vi "Autonomous Independent.vi"() -> ()   [LabVIEW 2020]
doc: "This VI is called when autonomous begins, and will automatically be terminated when autonomous ends. You can carry out timed or sensor driven robot movement independently without needing to return to the caller."
uses:
  <vilib>/Rock Robotics/WPI/ThirdParty/Phoenix-LabVIEW/Motor Controller/Controls/CTRE_Phoenix_MotorControl_ControlMode.ctl
  <vilib>/Rock Robotics/WPI/Solenoid/WPI_SolenoidValue.ctl
  <vilib>/Rock Robotics/WPI/Utilities/WPI_GetSetVariantRefNum.vi
  <vilib>/Rock Robotics/Network Tables/NT Read String.vi
  <vilib>/Rock Robotics/Network Tables/NT Write Numeric Array.vi
  <vilib>/Rock Robotics/WPI/Solenoid/WPI_SolenoidSetEnum.vi
  <vilib>/Rock Robotics/Network Tables/NT Read Number.vi
  AutonBoolean.vi
panel:
  out "Ty 24":dbl
  out "Ty 23":dbl
  out "Ty 22":dbl
  out "Ty 21":dbl
  out "Ty 20":dbl
  out "Ty 19":dbl
  out "Ty 18":dbl
  out "Ty 17":dbl
  out "Orange Limit Pressed 10":bool
  out "Blue Limit Pressed 10":bool
  out "Ty 16":dbl
  out "Orange Limit Pressed 9":bool
  out "Blue Limit Pressed 9":bool
  out "Ty 15":dbl
  out "Intake 5":bool
  out "Elevate 5":bool
  out "Ty 14":dbl
  out "Ty 13":dbl
  out "Ty 12":dbl
  out "Ty 11":dbl
  out "Ty 10":dbl
  out "Ty 9":dbl
  out "Orange Limit Pressed 4":bool
  out "Blue Limit Pressed 4":bool
  out "Ty 4":dbl
  out "Orange Limit Pressed 3":bool
  out "Blue Limit Pressed 3":bool
  out "Ty 3":dbl
  out "Intake 2":bool
  out "Elevate 2":bool
  out "Intake":bool
  out "Elevate":bool
  out "Orange Limit Pressed":bool
  out "Blue Limit Pressed":bool
  out "Ty":dbl
  out "Orange Limit Pressed 2":bool
  out "Blue Limit Pressed 2":bool
  out "Ty 2":dbl
  out "Intake 3":bool
  out "Elevate 3":bool
  out "Orange Limit Pressed 5":bool
  out "Blue Limit Pressed 5":bool
  out "Ty 5":dbl
  out "Orange Limit Pressed 6":bool
  out "Blue Limit Pressed 6":bool
  out "Ty 6":dbl
  out "Intake 4":bool
  out "Elevate 4":bool
  out "Orange Limit Pressed 7":bool
  out "Blue Limit Pressed 7":bool
  out "Ty 7":dbl
  out "Orange Limit Pressed 8":bool
  out "Blue Limit Pressed 8":bool
  out "Ty 8":dbl
  # "Be sure to right-click and choose Data Operations>>Make Current Value default if you want to save the array values with the VI"
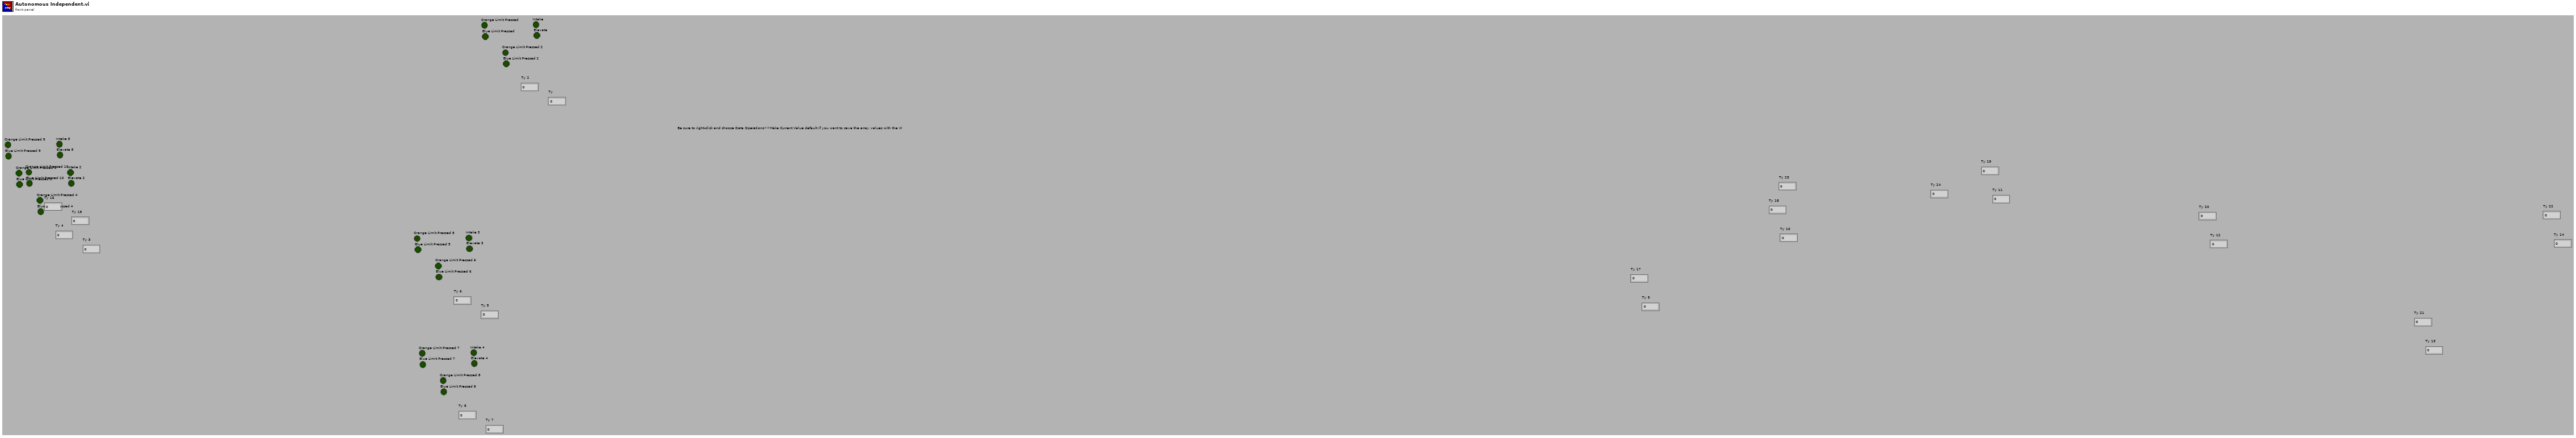
[diagram p1: front panel]
types:
  T1 = typedef "WPI_JoystickDevRef.ctl" = cluster{"Device":T2}
  T2 = typedef "WPI_JoystickDeviceEnum.ctl" = enum16{"USB 0", "USB 1", "USB 2", "USB 3", "USB 4", "USB 5"}
  T3 = typedef "WPI_SolenoidValue.ctl" = enum16{"Off", "On", "Forward", "Reverse"}
  T4 = typedef "WPI_SwitchDevRef.ctl" = cluster{"DevStatus":errorcluster, "DIO Channel":T5, "CntIndex":T6, "Normally Closed":bool}
  T5 = typedef "FPGA_DIOChannel.ctl" = enum8{"DIO 0", "DIO 1", "DIO 2", "DIO 3", "DIO 4", "DIO 5", "DIO 6", "DIO 7", "DIO 8", "DIO 9", "DIO MXP 0", "DIO MXP 1", "DIO MXP 2", "DIO MXP 3", "DIO MXP 4", "DIO MXP 5", "DIO MXP 6", "DIO MXP 7", "DIO MXP 8", "DIO MXP 9", "DIO MXP 10", "DIO MXP 11", "DIO MXP 12", "DIO MXP 13", "DIO MXP 14", "DIO MXP 15", "SPI Port CS1", "SPI Port CS2", "SPI Port CS3", "SPI Port MISO", "SPI Port MOSI", "Invalid"}
  T6 = typedef "FPGA_CounterCtrSystemIndex.ctl" = enum8{"Ctr 0", "Ctr 1", "Ctr 2", "Ctr 3", "Ctr 4", "Ctr 5", "Ctr 6", "Ctr 7", "Invalid"}
  T7 = typedef "WPI_SolenoidDevRef.ctl" = cluster{"DevStatus":errorcluster, "Pneumatics Control Module":u8, "Forward Solenoid Channel":T8, "Reverse Solenoid Channel":T8}
  T8 = typedef "WPI_SolenoidChannel.ctl" = enum8{"Solenoid 0", "Solenoid 1", "Solenoid 2", "Solenoid 3", "Solenoid 4", "Solenoid 5", "Solenoid 6", "Solenoid 7", "Solenoid 8", "Solenoid 9", "Solenoid 10", "Solenoid 11", "Solenoid 12", "Solenoid 13", "Solenoid 14", "Solenoid 15", "Invalid"}
  T9 = typedef "WPI_MotorControlDeviceRef.ctl" = cluster{"DeviceStatus":errorcluster, "Type":T10, "PWM":cluster{"PWM Channel":T11, "DeadBand":T12}, "CAN":cluster{"Device Number":u8, "SetOutput VI Ref":variant, "GetOutput VI Ref":variant, "Enable VI Ref":variant, "Disable VI Ref":variant, "Data":variant}, "Invert":bool, "DIO PWM":cluster{"PWM \"Enable\" Channel":T11, "DIOChannel":T5, "PWM Rate":dbl}}
  T10 = typedef "WPI_MotorControlType.ctl" = enum16{"PWM", "CAN", "DIO PWM"}
  T11 = typedef "FPGA_DIOPWMChannel.ctl" = enum8{"PWM 0", "PWM 1", "PWM 2", "PWM 3", "PWM 4", "PWM 5", "PWM 6", "PWM 7", "PWM 8", "PWM 9", "PWM MXP 0", "PWM MXP 1", "PWM MXP 2", "PWM MXP 3", "PWM MXP 4", "PWM MXP 5", "PWM MXP 6", "PWM MXP 7", "PWM MXP 8", "PWM MXP 9", "Invalid"}
  T12 = typedef "WPI_PWMDeadband.ctl" = cluster{"Name":string, "maxPositivePwm":i32, "minPositivePwm":i32, "centerPwm":i32, "maxNegativePwm":i32, "minNegativePwm":i32, "angularRange":u16}
  T13 = typedef "CTRE_Phoenix_MotorControl_ControlMode.ctl" = u16
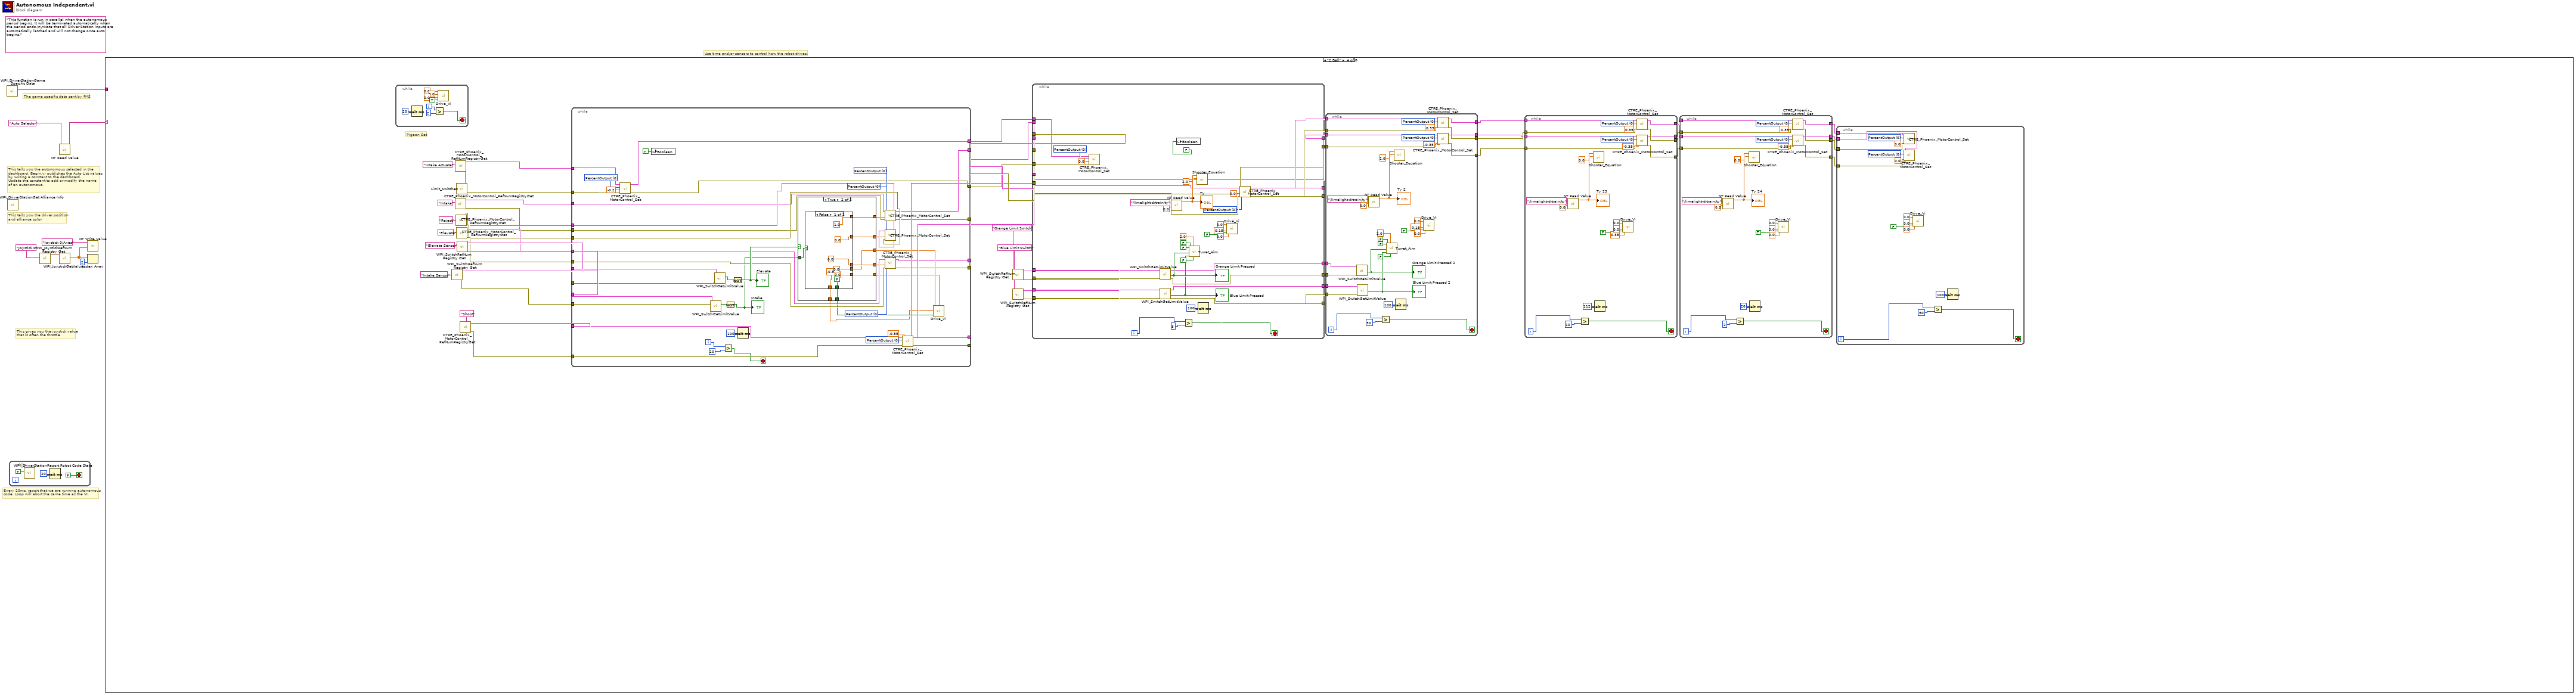
[diagram p0: block diagram]
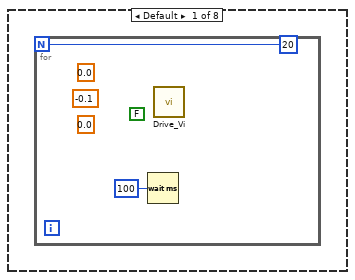
[diagram p2: hidden frame]
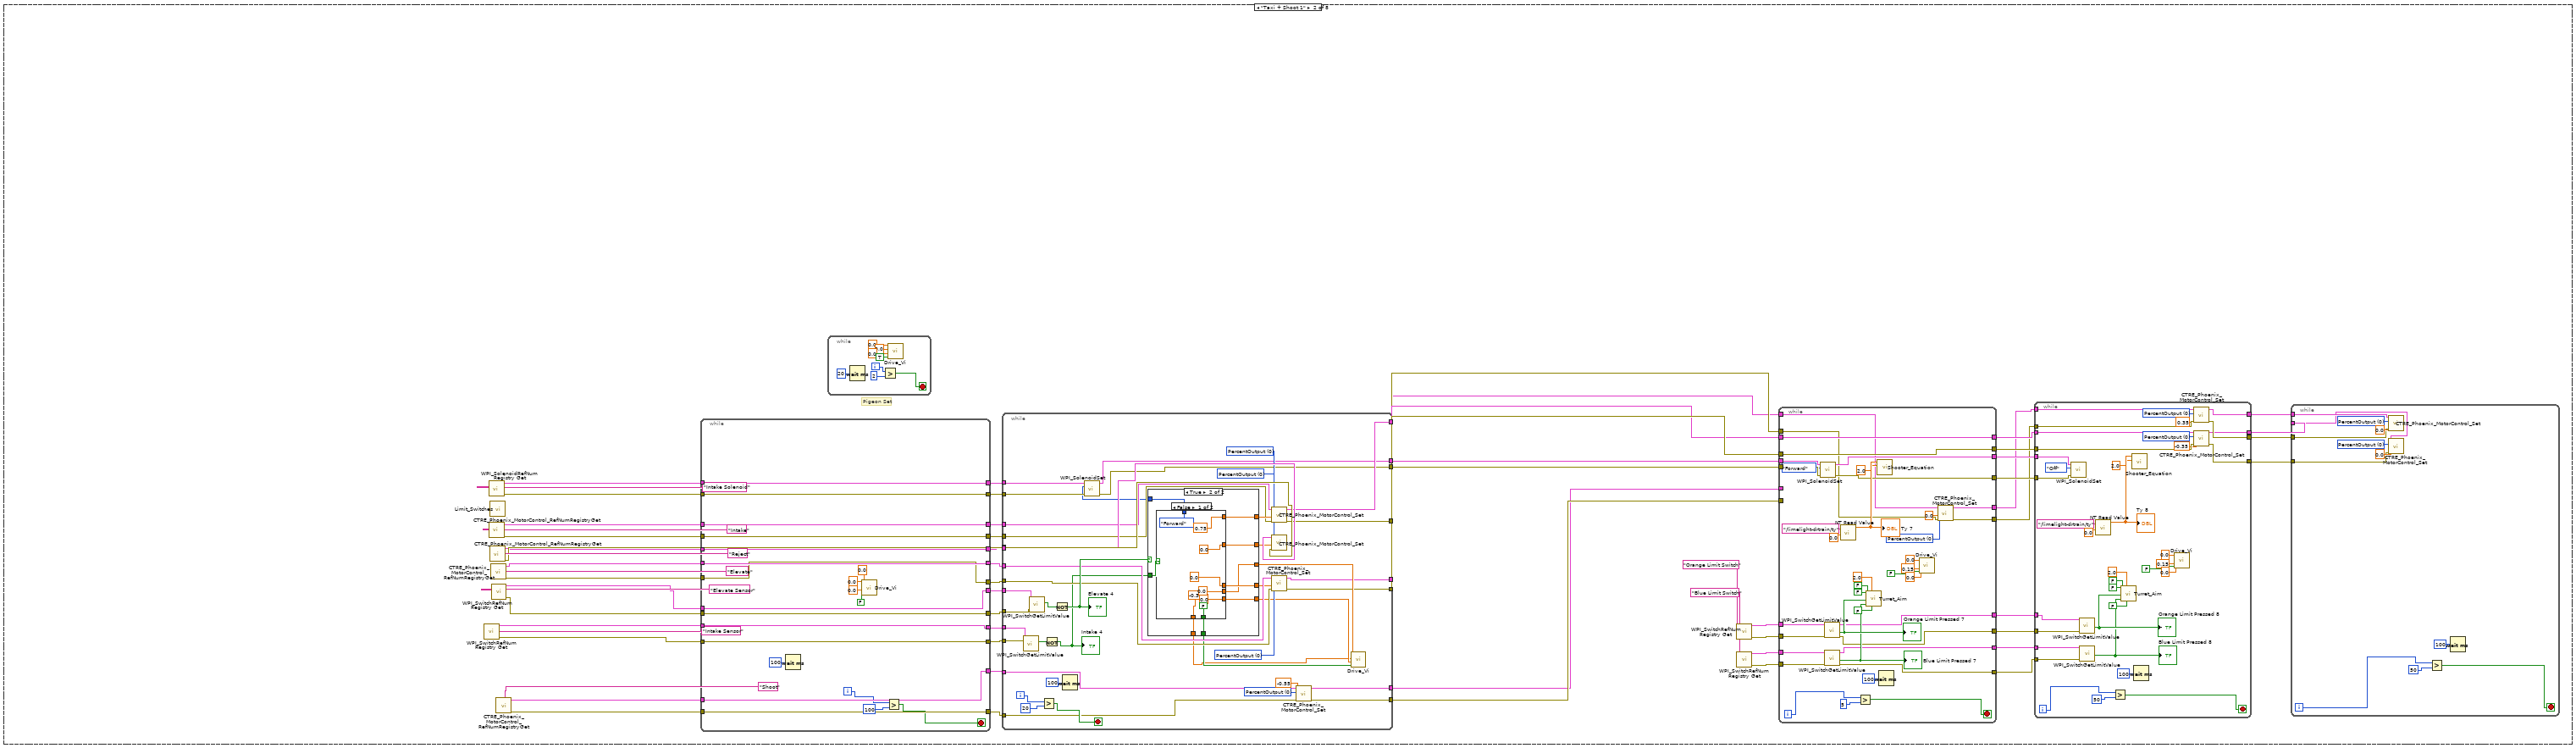
[diagram p3: hidden frame]
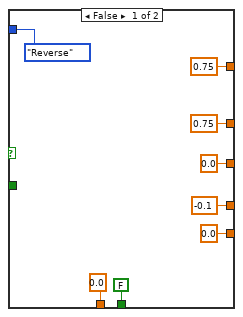
[diagram p4: hidden frame]
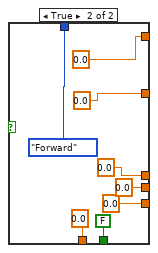
[diagram p5: hidden frame]
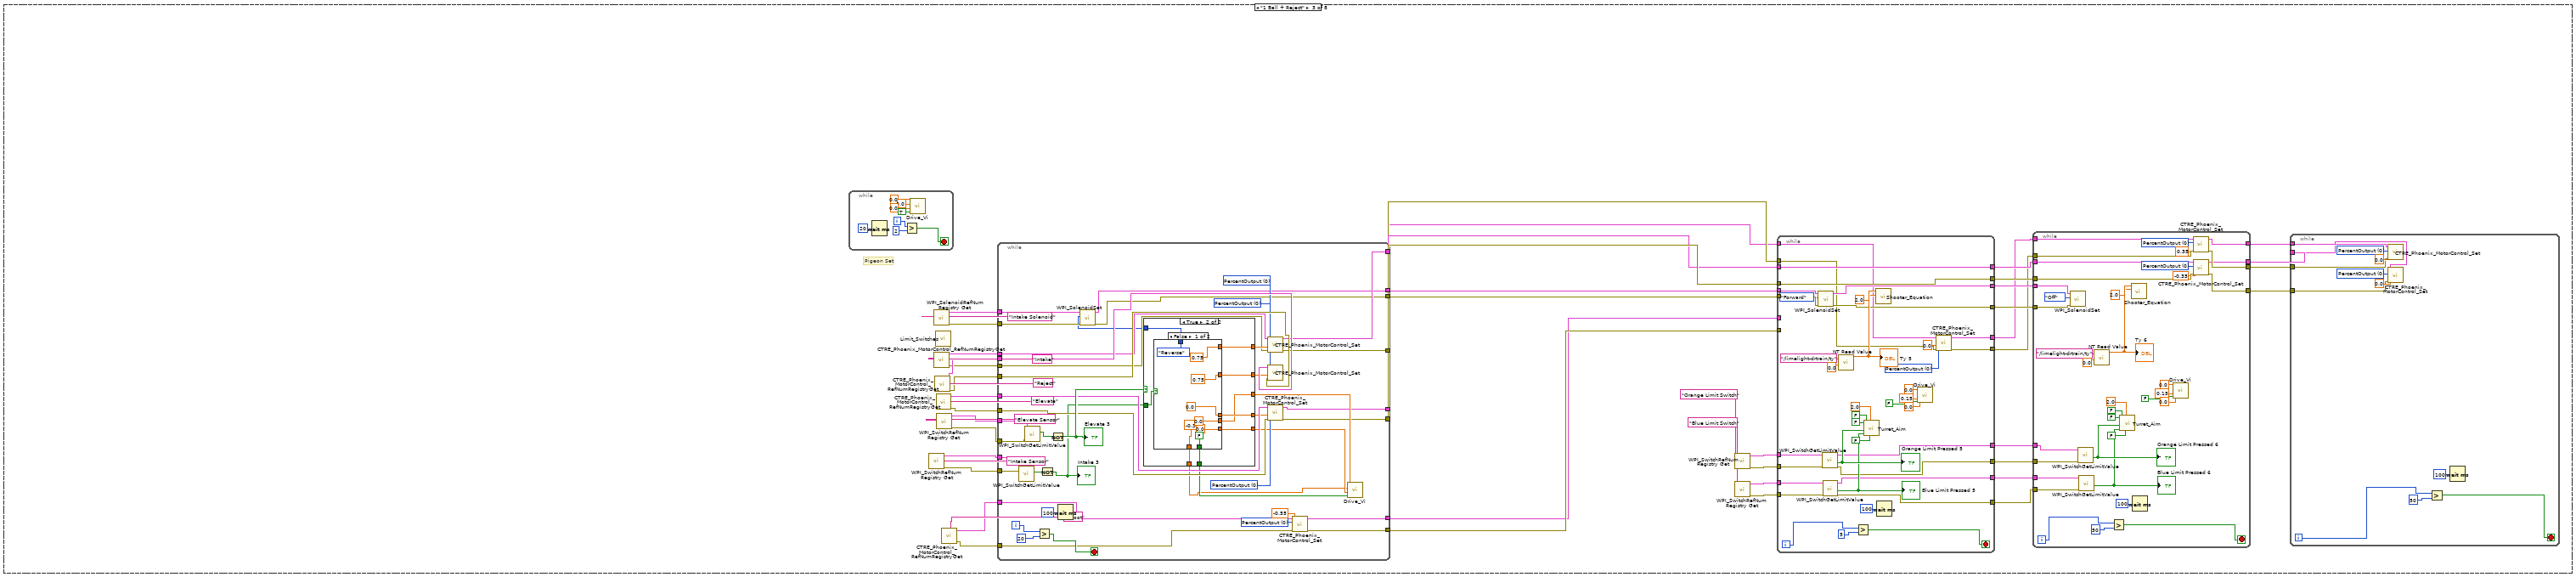
[diagram p6: hidden frame]
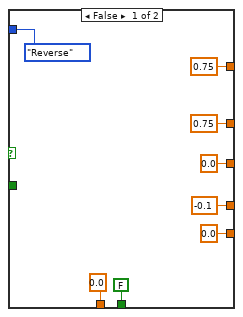
[diagram p7: hidden frame]
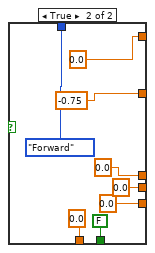
[diagram p8: hidden frame]
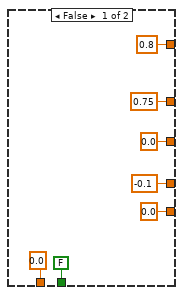
[diagram p9: hidden frame]
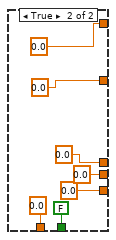
[diagram p10: hidden frame]
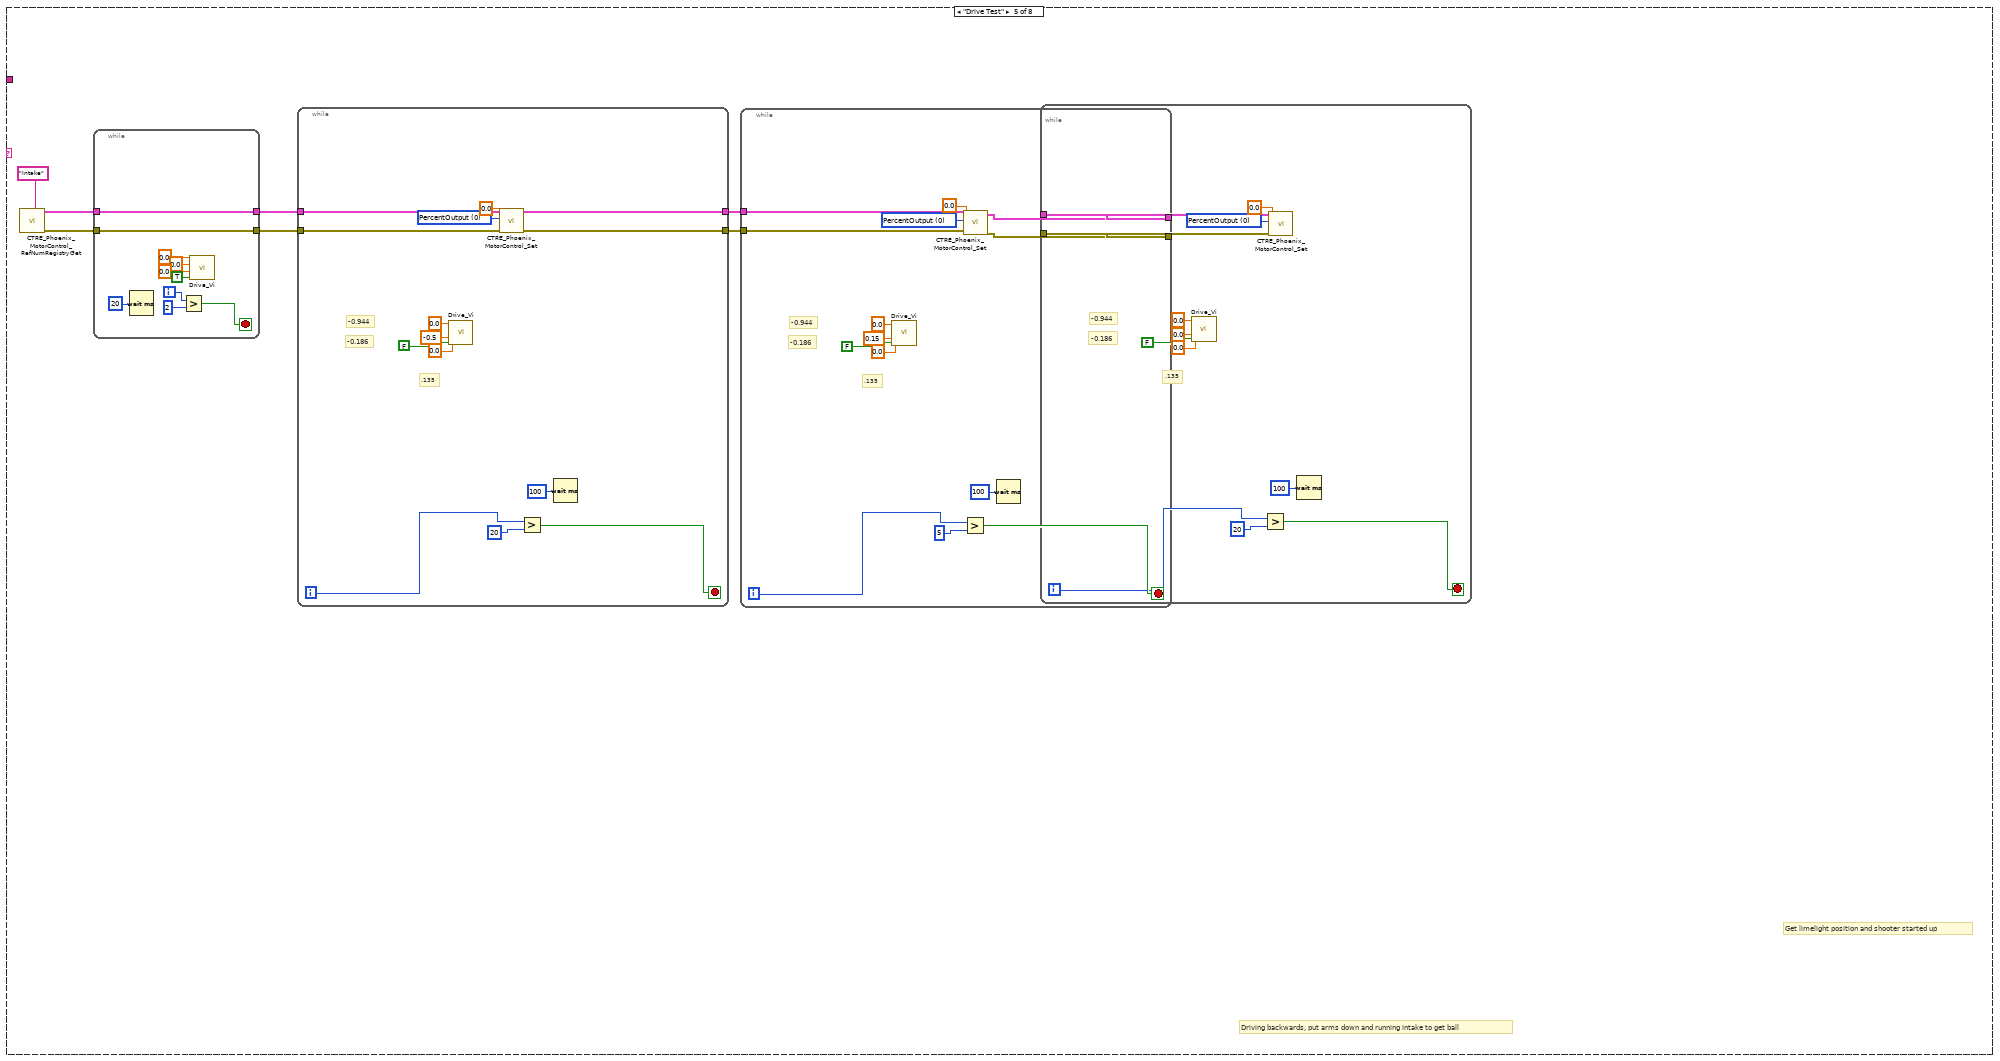
[diagram p11: hidden frame]
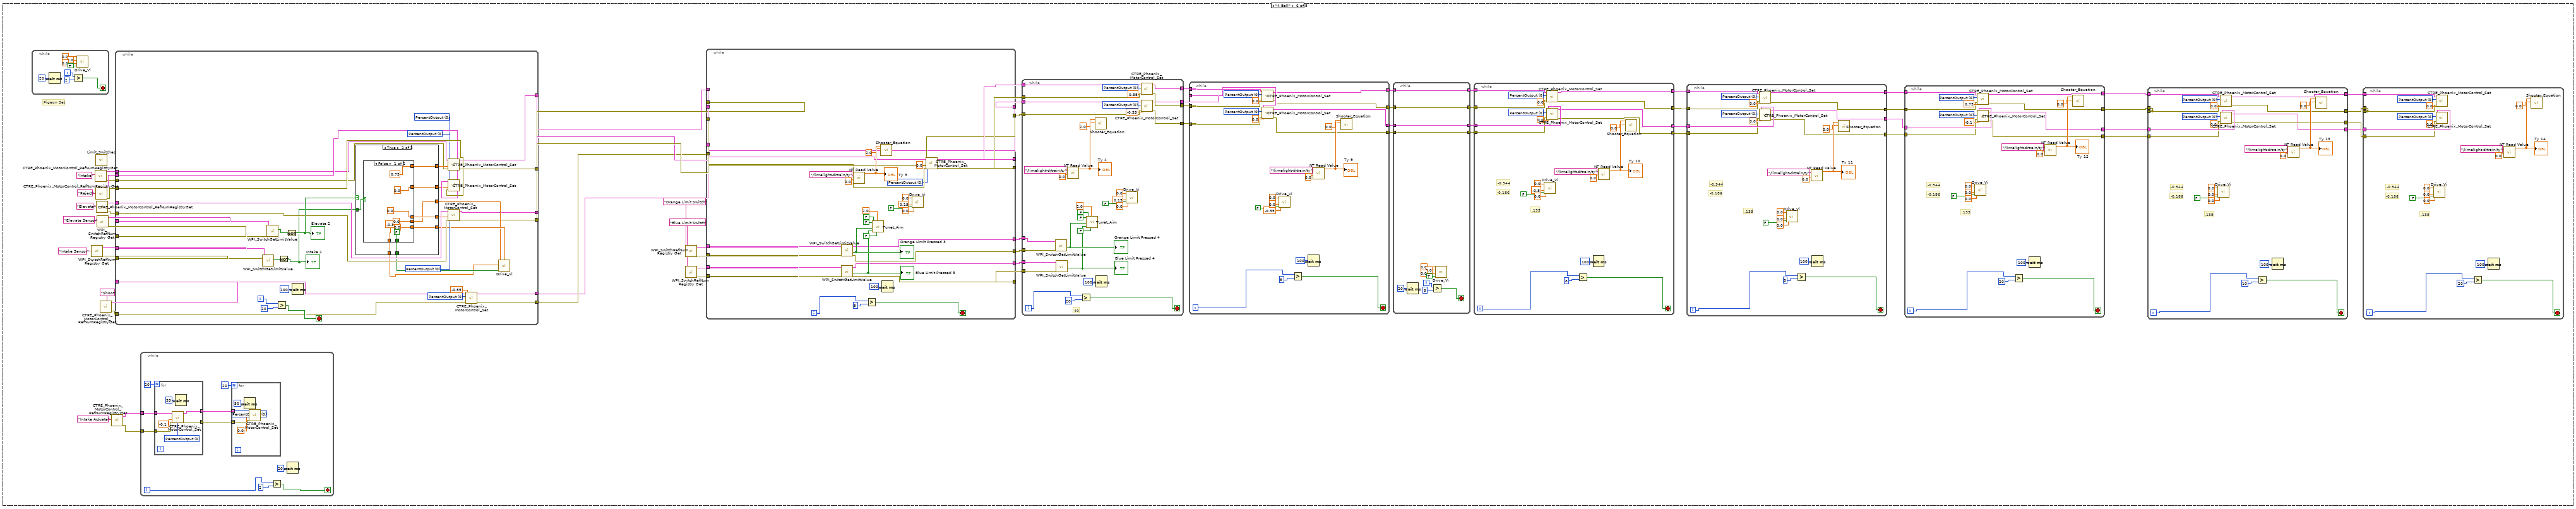
[diagram p12: hidden frame]
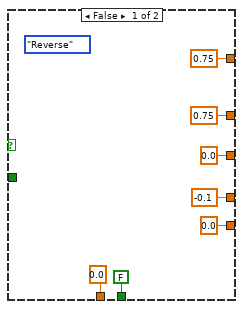
[diagram p13: hidden frame]
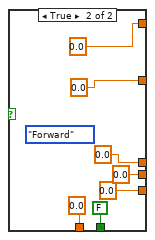
[diagram p14: hidden frame]
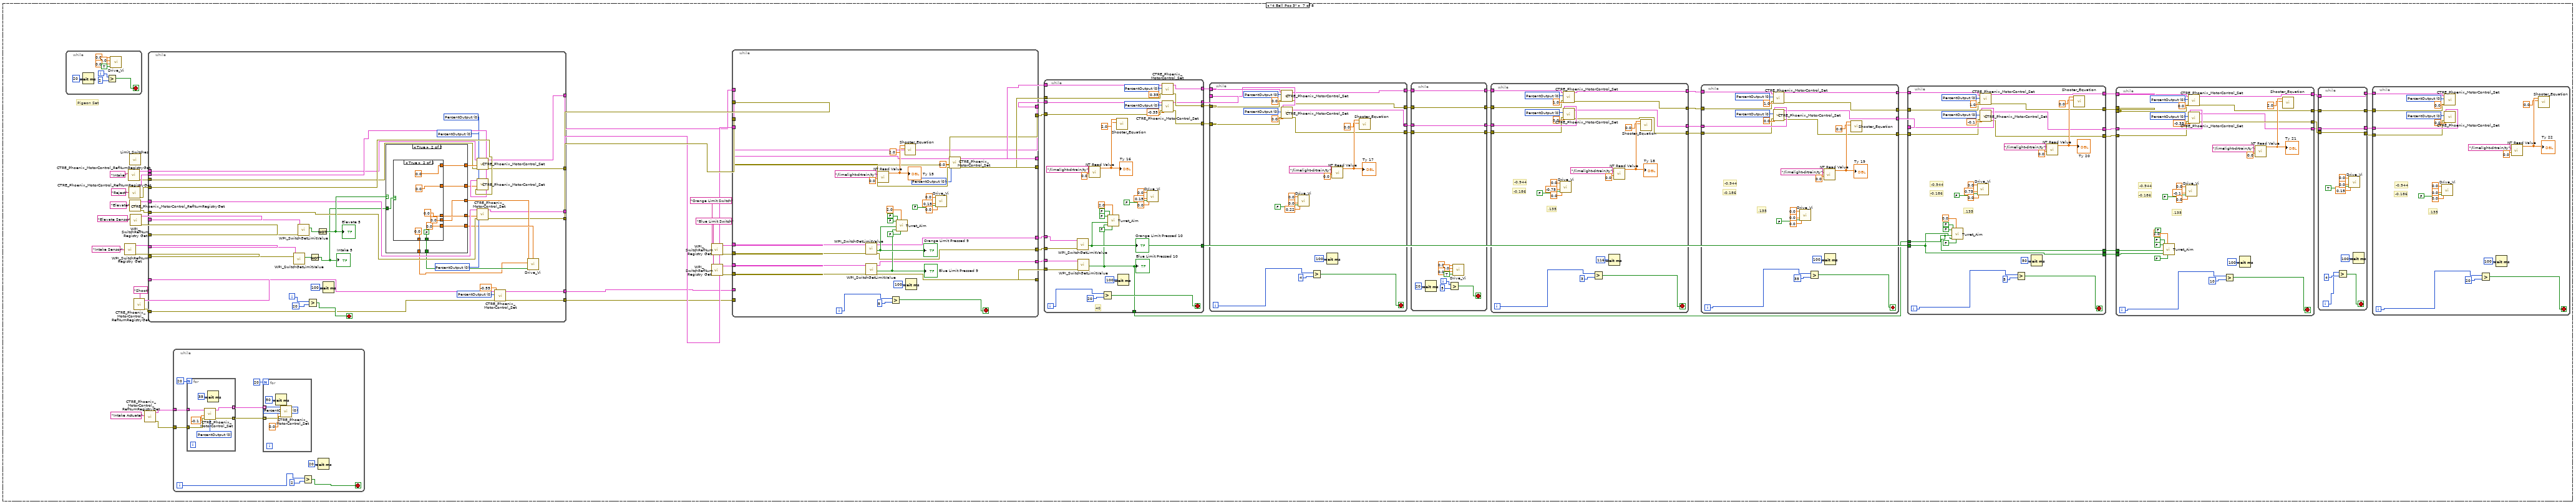
[diagram p15: hidden frame]
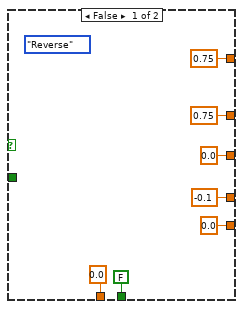
[diagram p16: hidden frame]
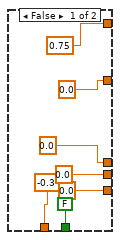
[diagram p17: hidden frame]
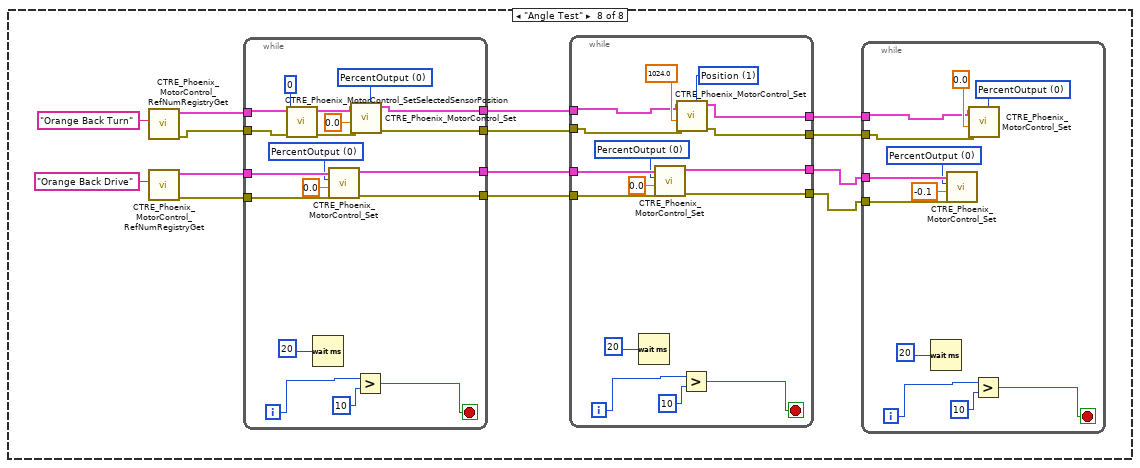
[diagram p18: hidden frame]
diagram:
  (unwired) "This function is run in parallel when the autonomous period begins. It will be terminated automatically when the period ends.\n\nNote that all Driver Station inputs are automatically latched and will not change once auto begins."
  # "The game specific data sent by FMS"
  # "This tells you the autonomous selected in the \ndashboard. Begin.vi publishes the Auto List values\nby writing a constant to the dashboard.\nUpdate the constant to add or modify the name\nof an autonomous."
  # "Every 20ms, report that we are running autonomous\ncode. Loop will abort the same time as the VI."
  # "This gives you the joystick value\nthat is often the throttle"
  # "Use time and/or sensors to control how the robot drives."
  # "This tells you the driver position\nand alliance color"
  n1 = call <vilib>:"WPI_DriverStationGame Specific Data.vi"() -> ("Game Specific Data"=w1:string)  [unwired: 11 in]
  n2 = call <vilib>:"WPI_DriverStationGet Alliance Info.vi"() -> ()  [unwired: 12 out]
  n3 = while {
    stop <- FALSE stop-if-true
    n4 = call <vilib>:"WPI_DriverStationReport Robot Code State.vi"("Autonomous"=TRUE) -> ()  [unwired: 10 in, 1 out]
    n5 = Wait (ms)(milliseconds to wait=u32 20) -> ()  [unwired: 1 out]
  }
  n6 = call <vilib>:"WPI_JoystickRefNum Registry Get.vi"("refnum name"="Joystick 0") -> ("JoystickDevRef"=w7:T1)  [unwired: 1 in, 9 out]
  n7 = call <vilib>:"WPI_JoystickGetValues.vi"("JoystickDevRef"=w7) -> ("Axes"=w3:dbl[])  [unwired: 6 in, 4 out]
  n8 = call-poly <vilib>:"NT Read Value.vi"("Name"="Auto Selector") -> ("String"=w4:string)  [unwired: 9 in, 1 out]
  n9 = call-poly <vilib>:"NT Write Value.vi"("Numeric Array"=w3, "Name"="Joystick 0/Axes") -> ()  [unwired: 9 in, 1 out]
  n10 = Index Array(array=w3, index=2) -> ()  [unwired: 1 out]
  n11 = case shown="\"2 Ball\"" w4 {
    tunnel: w1 -> [_ _ _ _ _ _ _ _]
    frame Default {
      n12 = for {
        N: 20 -> [_]
        (unwired) FALSE ("Middle Thumb")
        (unwired) 0.0 ("Z")
        (unwired) -0.1 ("Y")
        (unwired) 0.0 ("X")
        n13 = Wait (ms)(milliseconds to wait=u32 100) -> ()  [unwired: 1 out]
        n14 = call "Drive_Vi.vi"() -> ()  [unwired: 12 in]
      }
    }
    frame "Taxi + Shoot 1" {
      # "Pigeon Set"
      n15 = call <vilib>:"WPI_SwitchRefNum Registry Get.vi"("refnum name"="Intake Sensor") -> ("error out"=w18:errorcluster, "SwitchDevRef"=w20:T4)  [unwired: 9 in]
      n16 = call <vilib>:"WPI_SolenoidRefNum Registry Get.vi"("refnum name"="Intake Solenoid") -> ("error out"=w37:errorcluster, "SolenoidDevRef"=w39:T7)  [unwired: 9 in]
      n17 = call <vilib>:"CTRE_Phoenix_MotorControl_RefNumRegistryGet.vi"("refnum name"="Intake") -> ("error out"=w32:errorcluster, "PhoenixMotorControlDevRef"=w34:T9)  [unwired: 9 in]
      n18 = call <vilib>:"CTRE_Phoenix_MotorControl_RefNumRegistryGet.vi"("refnum name"="Reject") -> ("error out"=w68:errorcluster, "PhoenixMotorControlDevRef"=w30:T9)  [unwired: 9 in]
      n19 = call "Limit_Switches.vi"() -> ()  [unwired: 10 in, 2 out]
      n20 = call <vilib>:"CTRE_Phoenix_MotorControl_RefNumRegistryGet.vi"("refnum name"="Elevate") -> ("error out"=w26:errorcluster, "PhoenixMotorControlDevRef"=w28:T9)  [unwired: 9 in]
      n21 = call <vilib>:"WPI_SwitchRefNum Registry Get.vi"("refnum name"="Elevate Sensor") -> ("error out"=w22:errorcluster, "SwitchDevRef"=w24:T4)  [unwired: 9 in]
      n22 = call <vilib>:"CTRE_Phoenix_MotorControl_RefNumRegistryGet.vi"("refnum name"="Shoot") -> ("error out"=w14:errorcluster, "PhoenixMotorControlDevRef"=w17:T9)  [unwired: 9 in]
      n23 = while {
        tunnel: [w92] -> w38
        tunnel: w39 -> [w92]
        tunnel: [w91] -> w36
        tunnel: w37 -> [w91]
        tunnel: [w90] -> w35
        tunnel: w34 -> [w90]
        tunnel: [w89] -> w33
        tunnel: w32 -> [w89]
        tunnel: [w88] -> w31
        tunnel: w30 -> [w88]
        tunnel: [w87] -> w29
        tunnel: w28 -> [w87]
        tunnel: [w86] -> w27
        tunnel: w26 -> [w86]
        tunnel: [w85] -> w25
        tunnel: w24 -> [w85]
        tunnel: [w84] -> w23
        tunnel: w22 -> [w84]
        tunnel: [w83] -> w21
        tunnel: w20 -> [w83]
        tunnel: [w82] -> w19
        tunnel: w18 -> [w82]
        tunnel: [w81] -> w16
        tunnel: w17 -> [w81]
        tunnel: [w80] -> w15
        tunnel: w14 -> [w80]
        i -> [w76]
        stop <- w78 stop-if-true
        n24 = Wait (ms)(milliseconds to wait=u32 100) -> ()  [unwired: 1 out]
        n25 = call "Drive_Vi.vi"("Middle Thumb"=FALSE, "Z"=0.0, "Y"=0.0, "X"=0.0) -> ()  [unwired: 8 in]
        n26 = Greater?(x=w76, y=100) -> (0:w78:bool)
      }
      n27 = while {
        i -> [w266]
        stop <- w267 stop-if-true
        n28 = Wait (ms)(milliseconds to wait=u32 20) -> ()  [unwired: 1 out]
        n29 = Greater?(x=w266, y=2) -> (0:w267:bool)
        n30 = call "Drive_Vi.vi"("Middle Thumb"=TRUE, "Z"=0.0, "Y"=0.0, "X"=0.0) -> ()  [unwired: 8 in]
      }
      n31 = while {
        tunnel: w23 -> [w221]
        tunnel: w25 -> [w220]
        tunnel: w19 -> [w219]
        tunnel: w21 -> [w218]
        tunnel: w36 -> [w217]
        tunnel: w38 -> [w216]
        tunnel: w27 -> [w213]
        tunnel: w29 -> [w212]
        tunnel: w68 -> [w211]
        tunnel: w31 -> [w210]
        tunnel: w33 -> [w209]
        tunnel: w35 -> [w208]
        tunnel: [w196] -> w61
        tunnel: [w195] -> w60
        tunnel: [w194] -> w59
        tunnel: [w193] -> w58
        tunnel: w15 -> [w192]
        tunnel: w16 -> [w191]
        tunnel: [w188] -> w57
        tunnel: [w187] -> w56
        tunnel: [w186] -> w49
        tunnel: [w185] -> w48
        i -> [w224]
        stop <- w225 stop-if-true
        w190 = T13 0 items=["PercentOutput"=0, "Position"=1, "Velocity"=2, "Current"=3, "Follower"=5, "MotionProfile"=6, "MotionMagic"=7, "MotionProfileArc"=10, "Disabled"=15] ("Control Mode")
        w202 = T13 0 items=["PercentOutput"=0, "Position"=1, "Velocity"=2, "Current"=3, "Follower"=5, "MotionProfile"=6, "MotionMagic"=7, "MotionProfileArc"=10, "Disabled"=15] ("Control Mode")
        w203 = T13 0 items=["PercentOutput"=0, "Position"=1, "Velocity"=2, "Current"=3, "Follower"=5, "MotionProfile"=6, "MotionMagic"=7, "MotionProfileArc"=10, "Disabled"=15] ("Control Mode")
        w204 = T13 0 items=["PercentOutput"=0, "Position"=1, "Velocity"=2, "Current"=3, "Follower"=5, "MotionProfile"=6, "MotionMagic"=7, "MotionProfileArc"=10, "Disabled"=15] ("Control Mode")
        n32 = call <vilib>:"WPI_SwitchGetLimitValue.vi"("error in (no error)"=w219, "SwitchDevRef"=w218) -> ("Switch Pressed"=w222:bool)  [unwired: 7 in, 2 out]
        n33 = call <vilib>:"WPI_SwitchGetLimitValue.vi"("error in (no error)"=w221, "SwitchDevRef"=w220) -> ("Switch Pressed"=w223:bool)  [unwired: 7 in, 2 out]
        n34 = Greater?(x=w224, y=20) -> (0:w225:bool)
        n35 = Not(x=w222) -> (.not. x?=w207:bool)
        "Intake 4" <- w207
        n36 = Not(x=w223) -> (.not. x?=w215:bool)
        "Elevate 4" <- w215
        n37 = Wait (ms)(milliseconds to wait=u32 100) -> ()  [unwired: 1 out]
        n38 = case shown="True" w215 {
          tunnel: [0.75 ("Output") w244] -> w214
          tunnel: w207 -> [_ w241]
          tunnel: [0.75 ("Output") w243] -> w206
          tunnel: [-0.1 ("Output") w242] -> w205
          tunnel: [FALSE ("Middle Thumb") w240] -> w201
          tunnel: [0.0 ("Z") w239] -> w200
          tunnel: [0.0 ("Y") w238] -> w199
          tunnel: [0.0 ("X") w237] -> w198
          tunnel: [WPI_SolenoidValue."Reverse" ("Value") w236] -> w197
          frame False {
          }
          frame True {
            n39 = case shown="False" w241 {
              tunnel: [0.75 ("Output") 0.0 ("Output")] -> w244
              tunnel: [0.0 ("Output") 0.0 ("Output")] -> w243
              tunnel: [0.0 ("Output") 0.0 ("Output")] -> w242
              tunnel: [FALSE ("Middle Thumb") FALSE ("Middle Thumb")] -> w240
              tunnel: [0.0 ("Z") 0.0 ("Z")] -> w239
              tunnel: [-0.3 ("Y") 0.0 ("Y")] -> w238
              tunnel: [0.0 ("X") 0.0 ("X")] -> w237
              tunnel: [WPI_SolenoidValue."Forward" ("Value") WPI_SolenoidValue."Forward" ("Value")] -> w236
              frame False {
              }
              frame True {
              }
            }
          }
        }
        n40 = call-poly <vilib>:"WPI_SolenoidSet.vi"("error in (no error)"=w217, "Value"=w197, "SolenoidDevRef"=w216) -> ("error out"=w185:errorcluster, "SolenoidDevRef"=w186:T7)  [unwired: 7 in]
        n41 = call <vilib>:"CTRE_Phoenix_MotorControl_Set.vi"("error in (no error)"=w209, "Output"=w214, "Control Mode"=w202, "PhoenixMotorControlDevRef"=w208) -> ("error out"=w194:errorcluster, "PhoenixMotorControlDevRef"=w193:T9)  [unwired: 6 in]
        n42 = call <vilib>:"CTRE_Phoenix_MotorControl_Set.vi"("error in (no error)"=w211, "Output"=w206, "Control Mode"=w203, "PhoenixMotorControlDevRef"=w210) -> ()  [unwired: 6 in, 2 out]
        n43 = call <vilib>:"CTRE_Phoenix_MotorControl_Set.vi"("error in (no error)"=w213, "Output"=w205, "Control Mode"=w204, "PhoenixMotorControlDevRef"=w212) -> ("error out"=w196:errorcluster, "PhoenixMotorControlDevRef"=w195:T9)  [unwired: 6 in]
        n44 = call <vilib>:"CTRE_Phoenix_MotorControl_Set.vi"("error in (no error)"=w192, "Output"=-0.55, "Control Mode"=w190, "PhoenixMotorControlDevRef"=w191) -> ("error out"=w188:errorcluster, "PhoenixMotorControlDevRef"=w187:T9)  [unwired: 6 in]
        n45 = call "Drive_Vi.vi"("Middle Thumb"=w201, "Z"=w200, "Y"=w199, "X"=w198) -> ()  [unwired: 8 in]
      }
      n46 = call <vilib>:"WPI_SwitchRefNum Registry Get.vi"("refnum name"="Orange Limit Switch") -> ("error out"=w63:errorcluster, "SwitchDevRef"=w62:T4)  [unwired: 9 in]
      n47 = call <vilib>:"WPI_SwitchRefNum Registry Get.vi"("refnum name"="Blue Limit Switch") -> ("error out"=w65:errorcluster, "SwitchDevRef"=w64:T4)  [unwired: 9 in]
      n48 = while {
        tunnel: w57 -> [_]
        tunnel: w56 -> [_]
        tunnel: w65 -> [w182]
        tunnel: w64 -> [w181]
        tunnel: w63 -> [w180]
        tunnel: w62 -> [w179]
        tunnel: w61 -> [w158]
        tunnel: w60 -> [w157]
        tunnel: w59 -> [w148]
        tunnel: w58 -> [w149]
        tunnel: [w162] -> w55
        tunnel: [w161] -> w54
        tunnel: [w160] -> w53
        tunnel: [w159] -> w52
        tunnel: [w158] -> w51
        tunnel: [w157] -> w50
        tunnel: w49 -> [w156]
        tunnel: w48 -> [w155]
        tunnel: [w153] -> w47
        tunnel: [w152] -> w46
        tunnel: [w151] -> w45
        tunnel: [w150] -> w44
        i -> [w168]
        stop <- w167 stop-if-true
        w147 = T13 0 items=["PercentOutput"=0, "Position"=1, "Velocity"=2, "Current"=3, "Follower"=5, "MotionProfile"=6, "MotionMagic"=7, "MotionProfileArc"=10, "Disabled"=15] ("Control Mode")
        n49 = call-poly <vilib>:"WPI_SolenoidSet.vi"("error in (no error)"=w155, "Value"=WPI_SolenoidValue."Forward", "SolenoidDevRef"=w156) -> ("error out"=w152:errorcluster, "SolenoidDevRef"=w153:T7)  [unwired: 7 in]
        n50 = call <vilib>:"WPI_SwitchGetLimitValue.vi"("error in (no error)"=w180, "SwitchDevRef"=w179) -> ("error out"=w159:errorcluster, "Switch Pressed"=w178:bool, "SwitchDevRef"=w160:T4)  [unwired: 7 in]
        "Orange Limit Pressed 7" <- w178
        n51 = call <vilib>:"WPI_SwitchGetLimitValue.vi"("error in (no error)"=w182, "SwitchDevRef"=w181) -> ("error out"=w161:errorcluster, "Switch Pressed"=w177:bool, "SwitchDevRef"=w162:T4)  [unwired: 7 in]
        "Blue Limit Pressed 7" <- w177
        n52 = call-poly <vilib>:"NT Read Value.vi"("Default Value"=0.0, "Name"="/limelight-drtrain/ty") -> ("Numeric"=w172:dbl)  [unwired: 8 in, 1 out]
        "Ty 7" <- w172
        n53 = Greater?(x=w168, y=5) -> (0:w167:bool)
        n54 = call "Turret_Aim.vi"("View Button"=FALSE ("Driver Right Thumb"), "Left Trigger"=2.0, "Orange Limit Pressed"=w177, "Blue Limit Pressed"=w178, "Right Bumper"=FALSE, "Left Bumper"=FALSE) -> ()  [unwired: 6 in]
        n55 = call "Shooter_Equation.vi"("Right Trigger"=2.0, "Ty"=w172) -> ()  [unwired: 10 in]
        n56 = Wait (ms)(milliseconds to wait=u32 100) -> ()  [unwired: 1 out]
        n57 = call "Drive_Vi.vi"("Middle Thumb"=FALSE, "Z"=0.0, "Y"=0.15, "X"=0.0) -> ()  [unwired: 8 in]
        n58 = call <vilib>:"CTRE_Phoenix_MotorControl_Set.vi"("error in (no error)"=w148, "Output"=0.0, "Control Mode"=w147, "PhoenixMotorControlDevRef"=w149) -> ("error out"=w150:errorcluster, "PhoenixMotorControlDevRef"=w151:T9)  [unwired: 6 in]
      }
      n59 = while {
        tunnel: w54 -> [w143]
        tunnel: w55 -> [w142]
        tunnel: w52 -> [w141]
        tunnel: w51 -> [w128]
        tunnel: w50 -> [w127]
        tunnel: w44 -> [w126]
        tunnel: w45 -> [w125]
        tunnel: w53 -> [w116]
        tunnel: w47 -> [w115]
        tunnel: w46 -> [w114]
        tunnel: [w112] -> w43
        tunnel: [w111] -> w42
        tunnel: [w110] -> w41
        tunnel: [w109] -> w40
        i -> [w130]
        stop <- w129 stop-if-true
        w123 = T13 0 items=["PercentOutput"=0, "Position"=1, "Velocity"=2, "Current"=3, "Follower"=5, "MotionProfile"=6, "MotionMagic"=7, "MotionProfileArc"=10, "Disabled"=15] ("Control Mode")
        w124 = T13 0 items=["PercentOutput"=0, "Position"=1, "Velocity"=2, "Current"=3, "Follower"=5, "MotionProfile"=6, "MotionMagic"=7, "MotionProfileArc"=10, "Disabled"=15] ("Control Mode")
        n60 = call-poly <vilib>:"WPI_SolenoidSet.vi"("error in (no error)"=w114, "Value"=WPI_SolenoidValue."Off", "SolenoidDevRef"=w115) -> ()  [unwired: 7 in, 2 out]
        n61 = call <vilib>:"WPI_SwitchGetLimitValue.vi"("error in (no error)"=w141, "SwitchDevRef"=w116) -> ("Switch Pressed"=w140:bool)  [unwired: 7 in, 2 out]
        "Orange Limit Pressed 8" <- w140
        n62 = call <vilib>:"WPI_SwitchGetLimitValue.vi"("error in (no error)"=w143, "SwitchDevRef"=w142) -> ("Switch Pressed"=w139:bool)  [unwired: 7 in, 2 out]
        "Blue Limit Pressed 8" <- w139
        n63 = call-poly <vilib>:"NT Read Value.vi"("Default Value"=0.0, "Name"="/limelight-drtrain/ty") -> ("Numeric"=w134:dbl)  [unwired: 8 in, 1 out]
        "Ty 8" <- w134
        n64 = Greater?(x=w130, y=50) -> (0:w129:bool)
        n65 = call "Turret_Aim.vi"("View Button"=FALSE ("Driver Right Thumb"), "Left Trigger"=2.0, "Orange Limit Pressed"=w139, "Blue Limit Pressed"=w140, "Right Bumper"=FALSE, "Left Bumper"=FALSE) -> ()  [unwired: 6 in]
        n66 = call "Shooter_Equation.vi"("Right Trigger"=2.0, "Ty"=w134) -> ()  [unwired: 10 in]
        n67 = Wait (ms)(milliseconds to wait=u32 100) -> ()  [unwired: 1 out]
        n68 = call "Drive_Vi.vi"("Middle Thumb"=FALSE, "Z"=0.0, "Y"=0.15, "X"=0.0) -> ()  [unwired: 8 in]
        n69 = call <vilib>:"CTRE_Phoenix_MotorControl_Set.vi"("error in (no error)"=w126, "Output"=0.35, "Control Mode"=w123, "PhoenixMotorControlDevRef"=w125) -> ("error out"=w112:errorcluster, "PhoenixMotorControlDevRef"=w111:T9)  [unwired: 6 in]
        n70 = call <vilib>:"CTRE_Phoenix_MotorControl_Set.vi"("error in (no error)"=w128, "Output"=-0.35, "Control Mode"=w124, "PhoenixMotorControlDevRef"=w127) -> ("error out"=w109:errorcluster, "PhoenixMotorControlDevRef"=w110:T9)  [unwired: 6 in]
      }
      n71 = while {
        tunnel: w43 -> [w104]
        tunnel: w42 -> [w103]
        tunnel: w41 -> [w102]
        tunnel: w40 -> [w101]
        i -> [w99]
        stop <- w98 stop-if-true
        w107 = T13 0 items=["PercentOutput"=0, "Position"=1, "Velocity"=2, "Current"=3, "Follower"=5, "MotionProfile"=6, "MotionMagic"=7, "MotionProfileArc"=10, "Disabled"=15] ("Control Mode")
        w108 = T13 0 items=["PercentOutput"=0, "Position"=1, "Velocity"=2, "Current"=3, "Follower"=5, "MotionProfile"=6, "MotionMagic"=7, "MotionProfileArc"=10, "Disabled"=15] ("Control Mode")
        n72 = call <vilib>:"CTRE_Phoenix_MotorControl_Set.vi"("error in (no error)"=w104, "Output"=0.0, "Control Mode"=w107, "PhoenixMotorControlDevRef"=w103) -> ()  [unwired: 6 in, 2 out]
        n73 = call <vilib>:"CTRE_Phoenix_MotorControl_Set.vi"("error in (no error)"=w101, "Output"=0.0, "Control Mode"=w108, "PhoenixMotorControlDevRef"=w102) -> ()  [unwired: 6 in, 2 out]
        n74 = Greater?(x=w99, y=50) -> (0:w98:bool)
        n75 = Wait (ms)(milliseconds to wait=u32 100) -> ()  [unwired: 1 out]
      }
    }
    frame "1 Ball + Reject" {
      # "Pigeon Set"
      n76 = while {
        i -> [w487]
        stop <- w488 stop-if-true
        n77 = Wait (ms)(milliseconds to wait=u32 20) -> ()  [unwired: 1 out]
        n78 = Greater?(x=w487, y=2) -> (0:w488:bool)
        n79 = call "Drive_Vi.vi"("Middle Thumb"=TRUE, "Z"=0.0, "Y"=0.0, "X"=0.0) -> ()  [unwired: 8 in]
      }
      n80 = call <vilib>:"WPI_SwitchRefNum Registry Get.vi"("refnum name"="Intake Sensor") -> ("error out"=w308:errorcluster, "SwitchDevRef"=w307:T4)  [unwired: 9 in]
      n81 = call <vilib>:"WPI_SolenoidRefNum Registry Get.vi"("refnum name"="Intake Solenoid") -> ("error out"=w306:errorcluster, "SolenoidDevRef"=w305:T7)  [unwired: 9 in]
      n82 = call <vilib>:"CTRE_Phoenix_MotorControl_RefNumRegistryGet.vi"("refnum name"="Intake") -> ("error out"=w300:errorcluster, "PhoenixMotorControlDevRef"=w299:T9)  [unwired: 9 in]
      n83 = call <vilib>:"CTRE_Phoenix_MotorControl_RefNumRegistryGet.vi"("refnum name"="Reject") -> ("error out"=w302:errorcluster, "PhoenixMotorControlDevRef"=w301:T9)  [unwired: 9 in]
      n84 = call "Limit_Switches.vi"() -> ()  [unwired: 10 in, 2 out]
      n85 = call <vilib>:"CTRE_Phoenix_MotorControl_RefNumRegistryGet.vi"("refnum name"="Elevate") -> ("error out"=w304:errorcluster, "PhoenixMotorControlDevRef"=w303:T9)  [unwired: 9 in]
      n86 = call <vilib>:"WPI_SwitchRefNum Registry Get.vi"("refnum name"="Elevate Sensor") -> ("error out"=w310:errorcluster, "SwitchDevRef"=w309:T4)  [unwired: 9 in]
      n87 = call <vilib>:"CTRE_Phoenix_MotorControl_RefNumRegistryGet.vi"("refnum name"="Shoot") -> ("error out"=w288:errorcluster, "PhoenixMotorControlDevRef"=w287:T9)  [unwired: 9 in]
      n88 = while {
        tunnel: w310 -> [w442]
        tunnel: w309 -> [w441]
        tunnel: w308 -> [w440]
        tunnel: w307 -> [w439]
        tunnel: w306 -> [w438]
        tunnel: w305 -> [w437]
        tunnel: w304 -> [w434]
        tunnel: w303 -> [w433]
        tunnel: w302 -> [w432]
        tunnel: w301 -> [w431]
        tunnel: w300 -> [w430]
        tunnel: w299 -> [w429]
        tunnel: [w417] -> w292
        tunnel: [w416] -> w291
        tunnel: [w415] -> w290
        tunnel: [w414] -> w289
        tunnel: w288 -> [w413]
        tunnel: w287 -> [w412]
        tunnel: [w409] -> w286
        tunnel: [w408] -> w285
        tunnel: [w407] -> w278
        tunnel: [w406] -> w277
        i -> [w445]
        stop <- w446 stop-if-true
        w411 = T13 0 items=["PercentOutput"=0, "Position"=1, "Velocity"=2, "Current"=3, "Follower"=5, "MotionProfile"=6, "MotionMagic"=7, "MotionProfileArc"=10, "Disabled"=15] ("Control Mode")
        w423 = T13 0 items=["PercentOutput"=0, "Position"=1, "Velocity"=2, "Current"=3, "Follower"=5, "MotionProfile"=6, "MotionMagic"=7, "MotionProfileArc"=10, "Disabled"=15] ("Control Mode")
        w424 = T13 0 items=["PercentOutput"=0, "Position"=1, "Velocity"=2, "Current"=3, "Follower"=5, "MotionProfile"=6, "MotionMagic"=7, "MotionProfileArc"=10, "Disabled"=15] ("Control Mode")
        w425 = T13 0 items=["PercentOutput"=0, "Position"=1, "Velocity"=2, "Current"=3, "Follower"=5, "MotionProfile"=6, "MotionMagic"=7, "MotionProfileArc"=10, "Disabled"=15] ("Control Mode")
        n89 = call <vilib>:"WPI_SwitchGetLimitValue.vi"("error in (no error)"=w440, "SwitchDevRef"=w439) -> ("Switch Pressed"=w443:bool)  [unwired: 7 in, 2 out]
        n90 = call <vilib>:"WPI_SwitchGetLimitValue.vi"("error in (no error)"=w442, "SwitchDevRef"=w441) -> ("Switch Pressed"=w444:bool)  [unwired: 7 in, 2 out]
        n91 = Greater?(x=w445, y=20) -> (0:w446:bool)
        n92 = Not(x=w443) -> (.not. x?=w428:bool)
        "Intake 3" <- w428
        n93 = Not(x=w444) -> (.not. x?=w436:bool)
        "Elevate 3" <- w436
        n94 = Wait (ms)(milliseconds to wait=u32 100) -> ()  [unwired: 1 out]
        n95 = case shown="True" w436 {
          tunnel: [0.75 ("Output") w465] -> w435
          tunnel: w428 -> [_ w462]
          tunnel: [0.75 ("Output") w464] -> w427
          tunnel: [-0.1 ("Output") w463] -> w426
          tunnel: [FALSE ("Middle Thumb") w461] -> w422
          tunnel: [0.0 ("Z") w460] -> w421
          tunnel: [0.0 ("Y") w459] -> w420
          tunnel: [0.0 ("X") w458] -> w419
          tunnel: [WPI_SolenoidValue."Reverse" ("Value") w457] -> w418
          frame False {
          }
          frame True {
            n96 = case shown="False" w462 {
              tunnel: [0.75 ("Output") 0.0 ("Output")] -> w465
              tunnel: [0.75 ("Output") -0.75 ("Output")] -> w464
              tunnel: [0.0 ("Output") 0.0 ("Output")] -> w463
              tunnel: [FALSE ("Middle Thumb") FALSE ("Middle Thumb")] -> w461
              tunnel: [0.0 ("Z") 0.0 ("Z")] -> w460
              tunnel: [-0.3 ("Y") 0.0 ("Y")] -> w459
              tunnel: [0.0 ("X") 0.0 ("X")] -> w458
              tunnel: [WPI_SolenoidValue."Reverse" ("Value") WPI_SolenoidValue."Forward" ("Value")] -> w457
              frame False {
              }
              frame True {
              }
            }
          }
        }
        n97 = call-poly <vilib>:"WPI_SolenoidSet.vi"("error in (no error)"=w438, "Value"=w418, "SolenoidDevRef"=w437) -> ("error out"=w406:errorcluster, "SolenoidDevRef"=w407:T7)  [unwired: 7 in]
        n98 = call <vilib>:"CTRE_Phoenix_MotorControl_Set.vi"("error in (no error)"=w430, "Output"=w435, "Control Mode"=w423, "PhoenixMotorControlDevRef"=w429) -> ("error out"=w415:errorcluster, "PhoenixMotorControlDevRef"=w414:T9)  [unwired: 6 in]
        n99 = call <vilib>:"CTRE_Phoenix_MotorControl_Set.vi"("error in (no error)"=w432, "Output"=w427, "Control Mode"=w424, "PhoenixMotorControlDevRef"=w431) -> ()  [unwired: 6 in, 2 out]
        n100 = call <vilib>:"CTRE_Phoenix_MotorControl_Set.vi"("error in (no error)"=w434, "Output"=w426, "Control Mode"=w425, "PhoenixMotorControlDevRef"=w433) -> ("error out"=w417:errorcluster, "PhoenixMotorControlDevRef"=w416:T9)  [unwired: 6 in]
        n101 = call <vilib>:"CTRE_Phoenix_MotorControl_Set.vi"("error in (no error)"=w413, "Output"=-0.55, "Control Mode"=w411, "PhoenixMotorControlDevRef"=w412) -> ("error out"=w409:errorcluster, "PhoenixMotorControlDevRef"=w408:T9)  [unwired: 6 in]
        n102 = call "Drive_Vi.vi"("Middle Thumb"=w422, "Z"=w421, "Y"=w420, "X"=w419) -> ()  [unwired: 8 in]
      }
      n103 = call <vilib>:"WPI_SwitchRefNum Registry Get.vi"("refnum name"="Orange Limit Switch") -> ("error out"=w294:errorcluster, "SwitchDevRef"=w293:T4)  [unwired: 9 in]
      n104 = call <vilib>:"WPI_SwitchRefNum Registry Get.vi"("refnum name"="Blue Limit Switch") -> ("error out"=w296:errorcluster, "SwitchDevRef"=w295:T4)  [unwired: 9 in]
      n105 = while {
        tunnel: w286 -> [_]
        tunnel: w285 -> [_]
        tunnel: w296 -> [w403]
        tunnel: w295 -> [w402]
        tunnel: w294 -> [w401]
        tunnel: w293 -> [w400]
        tunnel: w292 -> [w379]
        tunnel: w291 -> [w378]
        tunnel: w290 -> [w369]
        tunnel: w289 -> [w370]
        tunnel: [w383] -> w284
        tunnel: [w382] -> w283
        tunnel: [w381] -> w282
        tunnel: [w380] -> w281
        tunnel: [w379] -> w280
        tunnel: [w378] -> w279
        tunnel: w278 -> [w377]
        tunnel: w277 -> [w376]
        tunnel: [w374] -> w276
        tunnel: [w373] -> w275
        tunnel: [w372] -> w274
        tunnel: [w371] -> w273
        i -> [w389]
        stop <- w388 stop-if-true
        w368 = T13 0 items=["PercentOutput"=0, "Position"=1, "Velocity"=2, "Current"=3, "Follower"=5, "MotionProfile"=6, "MotionMagic"=7, "MotionProfileArc"=10, "Disabled"=15] ("Control Mode")
        n106 = call-poly <vilib>:"WPI_SolenoidSet.vi"("error in (no error)"=w376, "Value"=WPI_SolenoidValue."Forward", "SolenoidDevRef"=w377) -> ("error out"=w373:errorcluster, "SolenoidDevRef"=w374:T7)  [unwired: 7 in]
        n107 = call <vilib>:"WPI_SwitchGetLimitValue.vi"("error in (no error)"=w401, "SwitchDevRef"=w400) -> ("error out"=w380:errorcluster, "Switch Pressed"=w399:bool, "SwitchDevRef"=w381:T4)  [unwired: 7 in]
        "Orange Limit Pressed 5" <- w399
        n108 = call <vilib>:"WPI_SwitchGetLimitValue.vi"("error in (no error)"=w403, "SwitchDevRef"=w402) -> ("error out"=w382:errorcluster, "Switch Pressed"=w398:bool, "SwitchDevRef"=w383:T4)  [unwired: 7 in]
        "Blue Limit Pressed 5" <- w398
        n109 = call-poly <vilib>:"NT Read Value.vi"("Default Value"=0.0, "Name"="/limelight-drtrain/ty") -> ("Numeric"=w393:dbl)  [unwired: 8 in, 1 out]
        "Ty 5" <- w393
        n110 = Greater?(x=w389, y=5) -> (0:w388:bool)
        n111 = call "Turret_Aim.vi"("View Button"=FALSE ("Driver Right Thumb"), "Left Trigger"=2.0, "Orange Limit Pressed"=w398, "Blue Limit Pressed"=w399, "Right Bumper"=FALSE, "Left Bumper"=FALSE) -> ()  [unwired: 6 in]
        n112 = call "Shooter_Equation.vi"("Right Trigger"=2.0, "Ty"=w393) -> ()  [unwired: 10 in]
        n113 = Wait (ms)(milliseconds to wait=u32 100) -> ()  [unwired: 1 out]
        n114 = call "Drive_Vi.vi"("Middle Thumb"=FALSE, "Z"=0.0, "Y"=0.15, "X"=0.0) -> ()  [unwired: 8 in]
        n115 = call <vilib>:"CTRE_Phoenix_MotorControl_Set.vi"("error in (no error)"=w369, "Output"=0.0, "Control Mode"=w368, "PhoenixMotorControlDevRef"=w370) -> ("error out"=w371:errorcluster, "PhoenixMotorControlDevRef"=w372:T9)  [unwired: 6 in]
      }
      n116 = while {
        tunnel: w283 -> [w364]
        tunnel: w284 -> [w363]
        tunnel: w281 -> [w362]
        tunnel: w280 -> [w349]
        tunnel: w279 -> [w348]
        tunnel: w273 -> [w347]
        tunnel: w274 -> [w346]
        tunnel: w282 -> [w337]
        tunnel: w276 -> [w336]
        tunnel: w275 -> [w335]
        tunnel: [w333] -> w272
        tunnel: [w332] -> w271
        tunnel: [w331] -> w270
        tunnel: [w330] -> w269
        i -> [w351]
        stop <- w350 stop-if-true
        w344 = T13 0 items=["PercentOutput"=0, "Position"=1, "Velocity"=2, "Current"=3, "Follower"=5, "MotionProfile"=6, "MotionMagic"=7, "MotionProfileArc"=10, "Disabled"=15] ("Control Mode")
        w345 = T13 0 items=["PercentOutput"=0, "Position"=1, "Velocity"=2, "Current"=3, "Follower"=5, "MotionProfile"=6, "MotionMagic"=7, "MotionProfileArc"=10, "Disabled"=15] ("Control Mode")
        n117 = call-poly <vilib>:"WPI_SolenoidSet.vi"("error in (no error)"=w335, "Value"=WPI_SolenoidValue."Off", "SolenoidDevRef"=w336) -> ()  [unwired: 7 in, 2 out]
        n118 = call <vilib>:"WPI_SwitchGetLimitValue.vi"("error in (no error)"=w362, "SwitchDevRef"=w337) -> ("Switch Pressed"=w361:bool)  [unwired: 7 in, 2 out]
        "Orange Limit Pressed 6" <- w361
        n119 = call <vilib>:"WPI_SwitchGetLimitValue.vi"("error in (no error)"=w364, "SwitchDevRef"=w363) -> ("Switch Pressed"=w360:bool)  [unwired: 7 in, 2 out]
        "Blue Limit Pressed 6" <- w360
        n120 = call-poly <vilib>:"NT Read Value.vi"("Default Value"=0.0, "Name"="/limelight-drtrain/ty") -> ("Numeric"=w355:dbl)  [unwired: 8 in, 1 out]
        "Ty 6" <- w355
        n121 = Greater?(x=w351, y=50) -> (0:w350:bool)
        n122 = call "Turret_Aim.vi"("View Button"=FALSE ("Driver Right Thumb"), "Left Trigger"=2.0, "Orange Limit Pressed"=w360, "Blue Limit Pressed"=w361, "Right Bumper"=FALSE, "Left Bumper"=FALSE) -> ()  [unwired: 6 in]
        n123 = call "Shooter_Equation.vi"("Right Trigger"=2.0, "Ty"=w355) -> ()  [unwired: 10 in]
        n124 = Wait (ms)(milliseconds to wait=u32 100) -> ()  [unwired: 1 out]
        n125 = call "Drive_Vi.vi"("Middle Thumb"=FALSE, "Z"=0.0, "Y"=0.15, "X"=0.0) -> ()  [unwired: 8 in]
        n126 = call <vilib>:"CTRE_Phoenix_MotorControl_Set.vi"("error in (no error)"=w347, "Output"=0.35, "Control Mode"=w344, "PhoenixMotorControlDevRef"=w346) -> ("error out"=w333:errorcluster, "PhoenixMotorControlDevRef"=w332:T9)  [unwired: 6 in]
        n127 = call <vilib>:"CTRE_Phoenix_MotorControl_Set.vi"("error in (no error)"=w349, "Output"=-0.35, "Control Mode"=w345, "PhoenixMotorControlDevRef"=w348) -> ("error out"=w330:errorcluster, "PhoenixMotorControlDevRef"=w331:T9)  [unwired: 6 in]
      }
      n128 = while {
        tunnel: w272 -> [w325]
        tunnel: w271 -> [w324]
        tunnel: w270 -> [w323]
        tunnel: w269 -> [w322]
        i -> [w320]
        stop <- w319 stop-if-true
        w328 = T13 0 items=["PercentOutput"=0, "Position"=1, "Velocity"=2, "Current"=3, "Follower"=5, "MotionProfile"=6, "MotionMagic"=7, "MotionProfileArc"=10, "Disabled"=15] ("Control Mode")
        w329 = T13 0 items=["PercentOutput"=0, "Position"=1, "Velocity"=2, "Current"=3, "Follower"=5, "MotionProfile"=6, "MotionMagic"=7, "MotionProfileArc"=10, "Disabled"=15] ("Control Mode")
        n129 = call <vilib>:"CTRE_Phoenix_MotorControl_Set.vi"("error in (no error)"=w325, "Output"=0.0, "Control Mode"=w328, "PhoenixMotorControlDevRef"=w324) -> ()  [unwired: 6 in, 2 out]
        n130 = call <vilib>:"CTRE_Phoenix_MotorControl_Set.vi"("error in (no error)"=w322, "Output"=0.0, "Control Mode"=w329, "PhoenixMotorControlDevRef"=w323) -> ()  [unwired: 6 in, 2 out]
        n131 = Greater?(x=w320, y=50) -> (0:w319:bool)
        n132 = Wait (ms)(milliseconds to wait=u32 100) -> ()  [unwired: 1 out]
      }
    }
    frame "2 Ball" {
      # "Pigeon Set"
      n133 = while {
        i -> [w761]
        stop <- w762 stop-if-true
        n134 = Wait (ms)(milliseconds to wait=u32 20) -> ()  [unwired: 1 out]
        n135 = Greater?(x=w761, y=2) -> (0:w762:bool)
        n136 = call "Drive_Vi.vi"("Middle Thumb"=TRUE, "Z"=0.0, "Y"=0.0, "X"=0.0) -> ()  [unwired: 8 in]
      }
      n137 = call <vilib>:"WPI_SwitchRefNum Registry Get.vi"("refnum name"="Intake Sensor") -> ("error out"=w536:errorcluster, "SwitchDevRef"=w535:T4)  [unwired: 9 in]
      n138 = call <vilib>:"CTRE_Phoenix_MotorControl_RefNumRegistryGet.vi"("refnum name"="Intake") -> ("error out"=w530:errorcluster, "PhoenixMotorControlDevRef"=w529:T9)  [unwired: 9 in]
      n139 = call <vilib>:"CTRE_Phoenix_MotorControl_RefNumRegistryGet.vi"("refnum name"="Intake Actuate") -> ("error out"=w505:errorcluster, "PhoenixMotorControlDevRef"=w504:T9)  [unwired: 9 in]
      n140 = call <vilib>:"CTRE_Phoenix_MotorControl_RefNumRegistryGet.vi"("refnum name"="Reject") -> ("error out"=w532:errorcluster, "PhoenixMotorControlDevRef"=w531:T9)  [unwired: 9 in]
      n141 = call "Limit_Switches.vi"() -> ()  [unwired: 10 in, 2 out]
      n142 = call <vilib>:"CTRE_Phoenix_MotorControl_RefNumRegistryGet.vi"("refnum name"="Elevate") -> ("error out"=w534:errorcluster, "PhoenixMotorControlDevRef"=w533:T9)  [unwired: 9 in]
      n143 = call <vilib>:"WPI_SwitchRefNum Registry Get.vi"("refnum name"="Elevate Sensor") -> ("error out"=w538:errorcluster, "SwitchDevRef"=w537:T4)  [unwired: 9 in]
      n144 = call <vilib>:"CTRE_Phoenix_MotorControl_RefNumRegistryGet.vi"("refnum name"="Shoot") -> ("error out"=w518:errorcluster, "PhoenixMotorControlDevRef"=w517:T9)  [unwired: 9 in]
      n145 = while {
        tunnel: w538 -> [w720]
        tunnel: w537 -> [w719]
        tunnel: w536 -> [w718]
        tunnel: w535 -> [w717]
        tunnel: w534 -> [w714]
        tunnel: w533 -> [w713]
        tunnel: w532 -> [w712]
        tunnel: w531 -> [w711]
        tunnel: w530 -> [w710]
        tunnel: w529 -> [w709]
        tunnel: [w698] -> w522
        tunnel: [w697] -> w521
        tunnel: [w696] -> w520
        tunnel: [w695] -> w519
        tunnel: w518 -> [w694]
        tunnel: w517 -> [w693]
        tunnel: [w690] -> w516
        tunnel: [w689] -> w515
        tunnel: w505 -> [w688]
        tunnel: w504 -> [w687]
        tunnel: [w684] -> w503
        tunnel: [w683] -> w502
        i -> [w723]
        stop <- w724 stop-if-true
        w686 = T13 0 items=["PercentOutput"=0, "Position"=1, "Velocity"=2, "Current"=3, "Follower"=5, "MotionProfile"=6, "MotionMagic"=7, "MotionProfileArc"=10, "Disabled"=15] ("Control Mode")
        w692 = T13 0 items=["PercentOutput"=0, "Position"=1, "Velocity"=2, "Current"=3, "Follower"=5, "MotionProfile"=6, "MotionMagic"=7, "MotionProfileArc"=10, "Disabled"=15] ("Control Mode")
        w703 = T13 0 items=["PercentOutput"=0, "Position"=1, "Velocity"=2, "Current"=3, "Follower"=5, "MotionProfile"=6, "MotionMagic"=7, "MotionProfileArc"=10, "Disabled"=15] ("Control Mode")
        w704 = T13 0 items=["PercentOutput"=0, "Position"=1, "Velocity"=2, "Current"=3, "Follower"=5, "MotionProfile"=6, "MotionMagic"=7, "MotionProfileArc"=10, "Disabled"=15] ("Control Mode")
        w705 = T13 0 items=["PercentOutput"=0, "Position"=1, "Velocity"=2, "Current"=3, "Follower"=5, "MotionProfile"=6, "MotionMagic"=7, "MotionProfileArc"=10, "Disabled"=15] ("Control Mode")
        n146 = call <vilib>:"CTRE_Phoenix_MotorControl_Set.vi"("error in (no error)"=w688, "Output"=-0.2, "Control Mode"=w686, "PhoenixMotorControlDevRef"=w687) -> ("error out"=w683:errorcluster, "PhoenixMotorControlDevRef"=w684:T9)  [unwired: 6 in]
        n147 = global write "AutonBoolean.vi" "Boolean"(TRUE ("Boolean")) -> ()
        n148 = call <vilib>:"WPI_SwitchGetLimitValue.vi"("error in (no error)"=w718, "SwitchDevRef"=w717) -> ("Switch Pressed"=w721:bool)  [unwired: 7 in, 2 out]
        n149 = call <vilib>:"WPI_SwitchGetLimitValue.vi"("error in (no error)"=w720, "SwitchDevRef"=w719) -> ("Switch Pressed"=w722:bool)  [unwired: 7 in, 2 out]
        n150 = Greater?(x=w723, y=20) -> (0:w724:bool)
        n151 = Not(x=w721) -> (.not. x?=w708:bool)
        "Intake" <- w708
        n152 = Not(x=w722) -> (.not. x?=w716:bool)
        "Elevate" <- w716
        n153 = Wait (ms)(milliseconds to wait=u32 100) -> ()  [unwired: 1 out]
        n154 = case shown="True" w716 {
          tunnel: [0.8 ("Output") w741] -> w715
          tunnel: w708 -> [_ w738]
          tunnel: [0.75 ("Output") w740] -> w707
          tunnel: [-0.1 ("Output") w739] -> w706
          tunnel: [FALSE ("Middle Thumb") w737] -> w702
          tunnel: [0.0 ("Z") w736] -> w701
          tunnel: [0.0 ("Y") w735] -> w700
          tunnel: [0.0 ("X") w734] -> w699
          frame False {
          }
          frame True {
            n155 = case shown="False" w738 {
              tunnel: [1.0 ("Output") 0.0 ("Output")] -> w741
              tunnel: [0.0 ("Output") 0.0 ("Output")] -> w740
              tunnel: [0.0 ("Output") 0.0 ("Output")] -> w739
              tunnel: [FALSE ("Middle Thumb") FALSE ("Middle Thumb")] -> w737
              tunnel: [0.0 ("Z") 0.0 ("Z")] -> w736
              tunnel: [-0.3 ("Y") 0.0 ("Y")] -> w735
              tunnel: [0.0 ("X") 0.0 ("X")] -> w734
              frame False {
              }
              frame True {
              }
            }
          }
        }
        n156 = call <vilib>:"CTRE_Phoenix_MotorControl_Set.vi"("error in (no error)"=w710, "Output"=w715, "Control Mode"=w703, "PhoenixMotorControlDevRef"=w709) -> ("error out"=w696:errorcluster, "PhoenixMotorControlDevRef"=w695:T9)  [unwired: 6 in]
        n157 = call <vilib>:"CTRE_Phoenix_MotorControl_Set.vi"("error in (no error)"=w712, "Output"=w707, "Control Mode"=w704, "PhoenixMotorControlDevRef"=w711) -> ()  [unwired: 6 in, 2 out]
        n158 = call <vilib>:"CTRE_Phoenix_MotorControl_Set.vi"("error in (no error)"=w714, "Output"=w706, "Control Mode"=w705, "PhoenixMotorControlDevRef"=w713) -> ("error out"=w698:errorcluster, "PhoenixMotorControlDevRef"=w697:T9)  [unwired: 6 in]
        n159 = call <vilib>:"CTRE_Phoenix_MotorControl_Set.vi"("error in (no error)"=w694, "Output"=-0.55, "Control Mode"=w692, "PhoenixMotorControlDevRef"=w693) -> ("error out"=w690:errorcluster, "PhoenixMotorControlDevRef"=w689:T9)  [unwired: 6 in]
        n160 = call "Drive_Vi.vi"("Middle Thumb"=w702, "Z"=w701, "Y"=w700, "X"=w699) -> ()  [unwired: 8 in]
      }
      n161 = call <vilib>:"WPI_SwitchRefNum Registry Get.vi"("refnum name"="Orange Limit Switch") -> ("error out"=w524:errorcluster, "SwitchDevRef"=w523:T4)  [unwired: 9 in]
      n162 = call <vilib>:"WPI_SwitchRefNum Registry Get.vi"("refnum name"="Blue Limit Switch") -> ("error out"=w526:errorcluster, "SwitchDevRef"=w525:T4)  [unwired: 9 in]
      n163 = while {
        tunnel: w516 -> [_]
        tunnel: w515 -> [_]
        tunnel: w526 -> [w679]
        tunnel: w525 -> [w678]
        tunnel: w524 -> [w677]
        tunnel: w523 -> [w676]
        tunnel: w522 -> [w655]
        tunnel: w521 -> [w654]
        tunnel: w520 -> [w650]
        tunnel: w519 -> [w651]
        tunnel: [w659] -> w514
        tunnel: [w658] -> w513
        tunnel: [w657] -> w512
        tunnel: [w656] -> w511
        tunnel: [w655] -> w510
        tunnel: [w654] -> w509
        tunnel: [w653] -> w508
        tunnel: [w652] -> w507
        tunnel: w503 -> [w645]
        tunnel: w502 -> [w644]
        i -> [w665]
        stop <- w664 stop-if-true
        w647 = T13 0 items=["PercentOutput"=0, "Position"=1, "Velocity"=2, "Current"=3, "Follower"=5, "MotionProfile"=6, "MotionMagic"=7, "MotionProfileArc"=10, "Disabled"=15] ("Control Mode")
        w649 = T13 0 items=["PercentOutput"=0, "Position"=1, "Velocity"=2, "Current"=3, "Follower"=5, "MotionProfile"=6, "MotionMagic"=7, "MotionProfileArc"=10, "Disabled"=15] ("Control Mode")
        n164 = call <vilib>:"CTRE_Phoenix_MotorControl_Set.vi"("error in (no error)"=w644, "Output"=0.0, "Control Mode"=w647, "PhoenixMotorControlDevRef"=w645) -> ()  [unwired: 6 in, 2 out]
        n165 = call <vilib>:"WPI_SwitchGetLimitValue.vi"("error in (no error)"=w677, "SwitchDevRef"=w676) -> ("error out"=w656:errorcluster, "Switch Pressed"=w675:bool, "SwitchDevRef"=w657:T4)  [unwired: 7 in]
        "Orange Limit Pressed" <- w675
        n166 = call <vilib>:"WPI_SwitchGetLimitValue.vi"("error in (no error)"=w679, "SwitchDevRef"=w678) -> ("error out"=w658:errorcluster, "Switch Pressed"=w674:bool, "SwitchDevRef"=w659:T4)  [unwired: 7 in]
        "Blue Limit Pressed" <- w674
        n167 = call-poly <vilib>:"NT Read Value.vi"("Default Value"=0.0, "Name"="/limelight-drtrain/ty") -> ("Numeric"=w669:dbl)  [unwired: 8 in, 1 out]
        "Ty" <- w669
        n168 = global write "AutonBoolean.vi" "Boolean"(FALSE ("Boolean")) -> ()
        n169 = Greater?(x=w665, y=5) -> (0:w664:bool)
        n170 = call "Turret_Aim.vi"("View Button"=FALSE ("Driver Right Thumb"), "Left Trigger"=2.0, "Orange Limit Pressed"=w674, "Blue Limit Pressed"=w675, "Right Bumper"=FALSE, "Left Bumper"=FALSE) -> ()  [unwired: 6 in]
        n171 = call "Shooter_Equation.vi"("Right Trigger"=2.0, "Ty"=w669) -> ()  [unwired: 10 in]
        n172 = Wait (ms)(milliseconds to wait=u32 100) -> ()  [unwired: 1 out]
        n173 = call "Drive_Vi.vi"("Middle Thumb"=FALSE, "Z"=0.0, "Y"=0.15, "X"=0.0) -> ()  [unwired: 8 in]
        n174 = call <vilib>:"CTRE_Phoenix_MotorControl_Set.vi"("error in (no error)"=w650, "Output"=0.0, "Control Mode"=w649, "PhoenixMotorControlDevRef"=w651) -> ("error out"=w652:errorcluster, "PhoenixMotorControlDevRef"=w653:T9)  [unwired: 6 in]
      }
      n175 = while {
        tunnel: w513 -> [w640]
        tunnel: w514 -> [w639]
        tunnel: w511 -> [w638]
        tunnel: w510 -> [w625]
        tunnel: w509 -> [w624]
        tunnel: w507 -> [w623]
        tunnel: w508 -> [w622]
        tunnel: w512 -> [w613]
        tunnel: [w612] -> w500
        tunnel: [w611] -> w501
        tunnel: [w610] -> w499
        tunnel: [w609] -> w498
        i -> [w627]
        stop <- w626 stop-if-true
        w620 = T13 0 items=["PercentOutput"=0, "Position"=1, "Velocity"=2, "Current"=3, "Follower"=5, "MotionProfile"=6, "MotionMagic"=7, "MotionProfileArc"=10, "Disabled"=15] ("Control Mode")
        w621 = T13 0 items=["PercentOutput"=0, "Position"=1, "Velocity"=2, "Current"=3, "Follower"=5, "MotionProfile"=6, "MotionMagic"=7, "MotionProfileArc"=10, "Disabled"=15] ("Control Mode")
        n176 = call <vilib>:"WPI_SwitchGetLimitValue.vi"("error in (no error)"=w638, "SwitchDevRef"=w613) -> ("Switch Pressed"=w637:bool)  [unwired: 7 in, 2 out]
        "Orange Limit Pressed 2" <- w637
        n177 = call <vilib>:"WPI_SwitchGetLimitValue.vi"("error in (no error)"=w640, "SwitchDevRef"=w639) -> ("Switch Pressed"=w636:bool)  [unwired: 7 in, 2 out]
        "Blue Limit Pressed 2" <- w636
        n178 = call-poly <vilib>:"NT Read Value.vi"("Default Value"=0.0, "Name"="/limelight-drtrain/ty") -> ("Numeric"=w631:dbl)  [unwired: 8 in, 1 out]
        "Ty 2" <- w631
        n179 = Greater?(x=w627, y=50) -> (0:w626:bool)
        n180 = call "Turret_Aim.vi"("View Button"=FALSE ("Driver Right Thumb"), "Left Trigger"=2.0, "Orange Limit Pressed"=w636, "Blue Limit Pressed"=w637, "Right Bumper"=FALSE, "Left Bumper"=FALSE) -> ()  [unwired: 6 in]
        n181 = call "Shooter_Equation.vi"("Right Trigger"=2.0, "Ty"=w631) -> ()  [unwired: 10 in]
        n182 = Wait (ms)(milliseconds to wait=u32 100) -> ()  [unwired: 1 out]
        n183 = call "Drive_Vi.vi"("Middle Thumb"=FALSE, "Z"=0.0, "Y"=0.15, "X"=0.0) -> ()  [unwired: 8 in]
        n184 = call <vilib>:"CTRE_Phoenix_MotorControl_Set.vi"("error in (no error)"=w623, "Output"=0.35, "Control Mode"=w620, "PhoenixMotorControlDevRef"=w622) -> ("error out"=w612:errorcluster, "PhoenixMotorControlDevRef"=w611:T9)  [unwired: 6 in]
        n185 = call <vilib>:"CTRE_Phoenix_MotorControl_Set.vi"("error in (no error)"=w625, "Output"=-0.35, "Control Mode"=w621, "PhoenixMotorControlDevRef"=w624) -> ("error out"=w609:errorcluster, "PhoenixMotorControlDevRef"=w610:T9)  [unwired: 6 in]
      }
      n186 = while {
        tunnel: w498 -> [w584]
        tunnel: w499 -> [w583]
        tunnel: w500 -> [w582]
        tunnel: w501 -> [w581]
        tunnel: [w572] -> w496
        tunnel: [w571] -> w497
        tunnel: [w570] -> w495
        tunnel: [w569] -> w494
        i -> [w586]
        stop <- w585 stop-if-true
        w579 = T13 0 items=["PercentOutput"=0, "Position"=1, "Velocity"=2, "Current"=3, "Follower"=5, "MotionProfile"=6, "MotionMagic"=7, "MotionProfileArc"=10, "Disabled"=15] ("Control Mode")
        w580 = T13 0 items=["PercentOutput"=0, "Position"=1, "Velocity"=2, "Current"=3, "Follower"=5, "MotionProfile"=6, "MotionMagic"=7, "MotionProfileArc"=10, "Disabled"=15] ("Control Mode")
        n187 = call-poly <vilib>:"NT Read Value.vi"("Default Value"=0.0, "Name"="/limelight-drtrain/ty") -> ("Numeric"=w590:dbl)  [unwired: 8 in, 1 out]
        "Ty 23" <- w590
        n188 = Greater?(x=w586, y=10) -> (0:w585:bool)
        n189 = call "Shooter_Equation.vi"("Right Trigger"=0.0, "Ty"=w590) -> ()  [unwired: 10 in]
        n190 = Wait (ms)(milliseconds to wait=u32 112) -> ()  [unwired: 1 out]
        n191 = call "Drive_Vi.vi"("Middle Thumb"=FALSE, "Z"=0.35, "Y"=0.0, "X"=0.0) -> ()  [unwired: 8 in]
        n192 = call <vilib>:"CTRE_Phoenix_MotorControl_Set.vi"("error in (no error)"=w582, "Output"=0.35, "Control Mode"=w579, "PhoenixMotorControlDevRef"=w581) -> ("error out"=w572:errorcluster, "PhoenixMotorControlDevRef"=w571:T9)  [unwired: 6 in]
        n193 = call <vilib>:"CTRE_Phoenix_MotorControl_Set.vi"("error in (no error)"=w584, "Output"=-0.35, "Control Mode"=w580, "PhoenixMotorControlDevRef"=w583) -> ("error out"=w569:errorcluster, "PhoenixMotorControlDevRef"=w570:T9)  [unwired: 6 in]
      }
      n194 = while {
        tunnel: w494 -> [w560]
        tunnel: w495 -> [w559]
        tunnel: w496 -> [w558]
        tunnel: w497 -> [w557]
        tunnel: [w548] -> w491
        tunnel: [w547] -> w493
        tunnel: [w546] -> w492
        tunnel: [w545] -> w490
        i -> [w562]
        stop <- w561 stop-if-true
        w555 = T13 0 items=["PercentOutput"=0, "Position"=1, "Velocity"=2, "Current"=3, "Follower"=5, "MotionProfile"=6, "MotionMagic"=7, "MotionProfileArc"=10, "Disabled"=15] ("Control Mode")
        w556 = T13 0 items=["PercentOutput"=0, "Position"=1, "Velocity"=2, "Current"=3, "Follower"=5, "MotionProfile"=6, "MotionMagic"=7, "MotionProfileArc"=10, "Disabled"=15] ("Control Mode")
        n195 = call-poly <vilib>:"NT Read Value.vi"("Default Value"=0.0, "Name"="/limelight-drtrain/ty") -> ("Numeric"=w566:dbl)  [unwired: 8 in, 1 out]
        "Ty 24" <- w566
        n196 = Greater?(x=w562, y=2) -> (0:w561:bool)
        n197 = call "Shooter_Equation.vi"("Right Trigger"=0.0, "Ty"=w566) -> ()  [unwired: 10 in]
        n198 = Wait (ms)(milliseconds to wait=u32 20) -> ()  [unwired: 1 out]
        n199 = call "Drive_Vi.vi"("Middle Thumb"=TRUE, "Z"=0.0, "Y"=0.0, "X"=0.0) -> ()  [unwired: 8 in]
        n200 = call <vilib>:"CTRE_Phoenix_MotorControl_Set.vi"("error in (no error)"=w558, "Output"=0.35, "Control Mode"=w555, "PhoenixMotorControlDevRef"=w557) -> ("error out"=w548:errorcluster, "PhoenixMotorControlDevRef"=w547:T9)  [unwired: 6 in]
        n201 = call <vilib>:"CTRE_Phoenix_MotorControl_Set.vi"("error in (no error)"=w560, "Output"=-0.35, "Control Mode"=w556, "PhoenixMotorControlDevRef"=w559) -> ("error out"=w545:errorcluster, "PhoenixMotorControlDevRef"=w546:T9)  [unwired: 6 in]
      }
      n202 = while {
        tunnel: w491 -> [w604]
        tunnel: w493 -> [w603]
        tunnel: w492 -> [w602]
        tunnel: w490 -> [w601]
        i -> [w599]
        stop <- w598 stop-if-true
        w607 = T13 0 items=["PercentOutput"=0, "Position"=1, "Velocity"=2, "Current"=3, "Follower"=5, "MotionProfile"=6, "MotionMagic"=7, "MotionProfileArc"=10, "Disabled"=15] ("Control Mode")
        w608 = T13 0 items=["PercentOutput"=0, "Position"=1, "Velocity"=2, "Current"=3, "Follower"=5, "MotionProfile"=6, "MotionMagic"=7, "MotionProfileArc"=10, "Disabled"=15] ("Control Mode")
        n203 = call <vilib>:"CTRE_Phoenix_MotorControl_Set.vi"("error in (no error)"=w604, "Output"=0.0, "Control Mode"=w607, "PhoenixMotorControlDevRef"=w603) -> ()  [unwired: 6 in, 2 out]
        n204 = call <vilib>:"CTRE_Phoenix_MotorControl_Set.vi"("error in (no error)"=w601, "Output"=0.0, "Control Mode"=w608, "PhoenixMotorControlDevRef"=w602) -> ()  [unwired: 6 in, 2 out]
        n205 = call "Drive_Vi.vi"("Middle Thumb"=FALSE, "Z"=0.0, "Y"=0.0, "X"=0.0) -> ()  [unwired: 8 in]
        n206 = Greater?(x=w599, y=50) -> (0:w598:bool)
        n207 = Wait (ms)(milliseconds to wait=u32 100) -> ()  [unwired: 1 out]
      }
    }
    frame "Drive Test" {
      # "Get limelight position and shooter started up"
      # "Driving backwards, put arms down and running intake to get ball"
      n208 = call <vilib>:"CTRE_Phoenix_MotorControl_RefNumRegistryGet.vi"("refnum name"="Intake") -> ("error out"=w765:errorcluster, "PhoenixMotorControlDevRef"=w767:T9)  [unwired: 9 in]
      n209 = while {
        tunnel: [w774] -> w766
        tunnel: w767 -> [w774]
        tunnel: [w773] -> w764
        tunnel: w765 -> [w773]
        i -> [w780]
        stop <- w781 stop-if-true
        n210 = Wait (ms)(milliseconds to wait=u32 20) -> ()  [unwired: 1 out]
        n211 = Greater?(x=w780, y=2) -> (0:w781:bool)
        n212 = call "Drive_Vi.vi"("Middle Thumb"=TRUE, "Z"=0.0, "Y"=0.0, "X"=0.0) -> ()  [unwired: 8 in]
      }
      n213 = while {
        tunnel: w766 -> [w814]
        tunnel: w764 -> [w813]
        tunnel: [w812] -> w771
        tunnel: [w811] -> w770
        i -> [w821]
        stop <- w820 stop-if-true
        w810 = T13 0 items=["PercentOutput"=0, "Position"=1, "Velocity"=2, "Current"=3, "Follower"=5, "MotionProfile"=6, "MotionMagic"=7, "MotionProfileArc"=10, "Disabled"=15] ("Control Mode")
        # "-0.186"
        # "-0.944"
        # ".135"
        n214 = call "Drive_Vi.vi"("Middle Thumb"=FALSE, "Z"=0.0, "Y"=-0.5, "X"=0.0) -> ()  [unwired: 8 in]
        n215 = call <vilib>:"CTRE_Phoenix_MotorControl_Set.vi"("error in (no error)"=w813, "Output"=0.0, "Control Mode"=w810, "PhoenixMotorControlDevRef"=w814) -> ("error out"=w811:errorcluster, "PhoenixMotorControlDevRef"=w812:T9)  [unwired: 6 in]
        n216 = Greater?(x=w821, y=20) -> (0:w820:bool)
        n217 = Wait (ms)(milliseconds to wait=u32 100) -> ()  [unwired: 1 out]
      }
      n218 = while {
        tunnel: w771 -> [w800]
        tunnel: w770 -> [w799]
        tunnel: [w798] -> w769
        tunnel: [w797] -> w768
        i -> [w807]
        stop <- w806 stop-if-true
        w796 = T13 0 items=["PercentOutput"=0, "Position"=1, "Velocity"=2, "Current"=3, "Follower"=5, "MotionProfile"=6, "MotionMagic"=7, "MotionProfileArc"=10, "Disabled"=15] ("Control Mode")
        # "-0.186"
        # "-0.944"
        # ".135"
        n219 = call "Drive_Vi.vi"("Middle Thumb"=FALSE, "Z"=0.0, "Y"=0.15, "X"=0.0) -> ()  [unwired: 8 in]
        n220 = Greater?(x=w807, y=5) -> (0:w806:bool)
        n221 = call <vilib>:"CTRE_Phoenix_MotorControl_Set.vi"("error in (no error)"=w799, "Output"=0.0, "Control Mode"=w796, "PhoenixMotorControlDevRef"=w800) -> ("error out"=w797:errorcluster, "PhoenixMotorControlDevRef"=w798:T9)  [unwired: 6 in]
        n222 = Wait (ms)(milliseconds to wait=u32 100) -> ()  [unwired: 1 out]
      }
      n223 = while {
        tunnel: w769 -> [w786]
        tunnel: w768 -> [w785]
        i -> [w793]
        stop <- w792 stop-if-true
        w784 = T13 0 items=["PercentOutput"=0, "Position"=1, "Velocity"=2, "Current"=3, "Follower"=5, "MotionProfile"=6, "MotionMagic"=7, "MotionProfileArc"=10, "Disabled"=15] ("Control Mode")
        # "-0.186"
        # "-0.944"
        # ".135"
        n224 = call "Drive_Vi.vi"("Middle Thumb"=FALSE, "Z"=0.0, "Y"=0.0, "X"=0.0) -> ()  [unwired: 8 in]
        n225 = Greater?(x=w793, y=20) -> (0:w792:bool)
        n226 = call <vilib>:"CTRE_Phoenix_MotorControl_Set.vi"("error in (no error)"=w785, "Output"=0.0, "Control Mode"=w784, "PhoenixMotorControlDevRef"=w786) -> ()  [unwired: 6 in, 2 out]
        n227 = Wait (ms)(milliseconds to wait=u32 100) -> ()  [unwired: 1 out]
      }
    }
    frame "4 Ball" {
      # "Pigeon Set"
      n228 = while {
        i -> [w1206]
        stop <- w1207 stop-if-true
        n229 = Wait (ms)(milliseconds to wait=u32 20) -> ()  [unwired: 1 out]
        n230 = Greater?(x=w1206, y=2) -> (0:w1207:bool)
        n231 = call "Drive_Vi.vi"("Middle Thumb"=TRUE, "Z"=0.0, "Y"=0.0, "X"=0.0) -> ()  [unwired: 8 in]
      }
      n232 = call <vilib>:"WPI_SwitchRefNum Registry Get.vi"("refnum name"="Intake Sensor") -> ("error out"=w883:errorcluster, "SwitchDevRef"=w882:T4)  [unwired: 9 in]
      n233 = call <vilib>:"CTRE_Phoenix_MotorControl_RefNumRegistryGet.vi"("refnum name"="Intake") -> ("error out"=w877:errorcluster, "PhoenixMotorControlDevRef"=w876:T9)  [unwired: 9 in]
      n234 = call <vilib>:"CTRE_Phoenix_MotorControl_RefNumRegistryGet.vi"("refnum name"="Reject") -> ("error out"=w879:errorcluster, "PhoenixMotorControlDevRef"=w878:T9)  [unwired: 9 in]
      n235 = call "Limit_Switches.vi"() -> ()  [unwired: 10 in, 2 out]
      n236 = call <vilib>:"CTRE_Phoenix_MotorControl_RefNumRegistryGet.vi"("refnum name"="Elevate") -> ("error out"=w881:errorcluster, "PhoenixMotorControlDevRef"=w880:T9)  [unwired: 9 in]
      n237 = call <vilib>:"WPI_SwitchRefNum Registry Get.vi"("refnum name"="Elevate Sensor") -> ("error out"=w885:errorcluster, "SwitchDevRef"=w884:T4)  [unwired: 9 in]
      n238 = call <vilib>:"CTRE_Phoenix_MotorControl_RefNumRegistryGet.vi"("refnum name"="Shoot") -> ("error out"=w865:errorcluster, "PhoenixMotorControlDevRef"=w864:T9)  [unwired: 9 in]
      n239 = call <vilib>:"CTRE_Phoenix_MotorControl_RefNumRegistryGet.vi"("refnum name"="Intake Actuate") -> ("error out"=w831:errorcluster, "PhoenixMotorControlDevRef"=w832:T9)  [unwired: 9 in]
      n240 = while {
        tunnel: w885 -> [w1165]
        tunnel: w884 -> [w1164]
        tunnel: w883 -> [w1163]
        tunnel: w882 -> [w1162]
        tunnel: w881 -> [w1159]
        tunnel: w880 -> [w1158]
        tunnel: w879 -> [w1157]
        tunnel: w878 -> [w1156]
        tunnel: w877 -> [w1155]
        tunnel: w876 -> [w1154]
        tunnel: [w1143] -> w869
        tunnel: [w1142] -> w868
        tunnel: [w1141] -> w867
        tunnel: [w1140] -> w866
        tunnel: w865 -> [w1139]
        tunnel: w864 -> [w1138]
        tunnel: [w1135] -> w863
        tunnel: [w1134] -> w862
        i -> [w1168]
        stop <- w1169 stop-if-true
        w1137 = T13 0 items=["PercentOutput"=0, "Position"=1, "Velocity"=2, "Current"=3, "Follower"=5, "MotionProfile"=6, "MotionMagic"=7, "MotionProfileArc"=10, "Disabled"=15] ("Control Mode")
        w1148 = T13 0 items=["PercentOutput"=0, "Position"=1, "Velocity"=2, "Current"=3, "Follower"=5, "MotionProfile"=6, "MotionMagic"=7, "MotionProfileArc"=10, "Disabled"=15] ("Control Mode")
        w1149 = T13 0 items=["PercentOutput"=0, "Position"=1, "Velocity"=2, "Current"=3, "Follower"=5, "MotionProfile"=6, "MotionMagic"=7, "MotionProfileArc"=10, "Disabled"=15] ("Control Mode")
        w1150 = T13 0 items=["PercentOutput"=0, "Position"=1, "Velocity"=2, "Current"=3, "Follower"=5, "MotionProfile"=6, "MotionMagic"=7, "MotionProfileArc"=10, "Disabled"=15] ("Control Mode")
        n241 = call <vilib>:"WPI_SwitchGetLimitValue.vi"("error in (no error)"=w1163, "SwitchDevRef"=w1162) -> ("Switch Pressed"=w1166:bool)  [unwired: 7 in, 2 out]
        n242 = call <vilib>:"WPI_SwitchGetLimitValue.vi"("error in (no error)"=w1165, "SwitchDevRef"=w1164) -> ("Switch Pressed"=w1167:bool)  [unwired: 7 in, 2 out]
        n243 = Greater?(x=w1168, y=20) -> (0:w1169:bool)
        n244 = Not(x=w1166) -> (.not. x?=w1153:bool)
        "Intake 2" <- w1153
        n245 = Not(x=w1167) -> (.not. x?=w1161:bool)
        "Elevate 2" <- w1161
        n246 = Wait (ms)(milliseconds to wait=u32 100) -> ()  [unwired: 1 out]
        n247 = case shown="True" w1161 {
          tunnel: [0.75 ("Output") w1186] -> w1160
          tunnel: w1153 -> [_ w1183]
          tunnel: [0.75 ("Output") w1185] -> w1152
          tunnel: [-0.1 ("Output") w1184] -> w1151
          tunnel: [FALSE ("Middle Thumb") w1182] -> w1147
          tunnel: [0.0 ("Z") w1181] -> w1146
          tunnel: [0.0 ("Y") w1180] -> w1145
          tunnel: [0.0 ("X") w1179] -> w1144
          frame False {
            (unwired) WPI_SolenoidValue."Reverse" ("Value")
          }
          frame True {
            n248 = case shown="False" w1183 {
              tunnel: [0.75 ("Output") 0.0 ("Output")] -> w1186
              tunnel: [0.0 ("Output") 0.0 ("Output")] -> w1185
              tunnel: [0.0 ("Output") 0.0 ("Output")] -> w1184
              tunnel: [FALSE ("Middle Thumb") FALSE ("Middle Thumb")] -> w1182
              tunnel: [0.0 ("Z") 0.0 ("Z")] -> w1181
              tunnel: [-0.3 ("Y") 0.0 ("Y")] -> w1180
              tunnel: [0.0 ("X") 0.0 ("X")] -> w1179
              frame False {
              }
              frame True {
                (unwired) WPI_SolenoidValue."Forward" ("Value")
              }
            }
          }
        }
        n249 = call <vilib>:"CTRE_Phoenix_MotorControl_Set.vi"("error in (no error)"=w1155, "Output"=w1160, "Control Mode"=w1148, "PhoenixMotorControlDevRef"=w1154) -> ("error out"=w1141:errorcluster, "PhoenixMotorControlDevRef"=w1140:T9)  [unwired: 6 in]
        n250 = call <vilib>:"CTRE_Phoenix_MotorControl_Set.vi"("error in (no error)"=w1157, "Output"=w1152, "Control Mode"=w1149, "PhoenixMotorControlDevRef"=w1156) -> ()  [unwired: 6 in, 2 out]
        n251 = call <vilib>:"CTRE_Phoenix_MotorControl_Set.vi"("error in (no error)"=w1159, "Output"=w1151, "Control Mode"=w1150, "PhoenixMotorControlDevRef"=w1158) -> ("error out"=w1143:errorcluster, "PhoenixMotorControlDevRef"=w1142:T9)  [unwired: 6 in]
        n252 = call <vilib>:"CTRE_Phoenix_MotorControl_Set.vi"("error in (no error)"=w1139, "Output"=-0.55, "Control Mode"=w1137, "PhoenixMotorControlDevRef"=w1138) -> ("error out"=w1135:errorcluster, "PhoenixMotorControlDevRef"=w1134:T9)  [unwired: 6 in]
        n253 = call "Drive_Vi.vi"("Middle Thumb"=w1147, "Z"=w1146, "Y"=w1145, "X"=w1144) -> ()  [unwired: 8 in]
      }
      n254 = while {
        tunnel: w832 -> [w913]
        tunnel: w831 -> [w912]
        i -> [w905]
        stop <- w904 stop-if-true
        n255 = for {
          N: 20 -> [_]
          tunnel: w913 -> [w925]
          tunnel: w912 -> [w924]
          tunnel: [w923] -> w911 mode=indexing
          tunnel: [w922] -> w910 mode=indexing
          w920 = T13 0 items=["PercentOutput"=0, "Position"=1, "Velocity"=2, "Current"=3, "Follower"=5, "MotionProfile"=6, "MotionMagic"=7, "MotionProfileArc"=10, "Disabled"=15] ("Control Mode")
          n256 = call <vilib>:"CTRE_Phoenix_MotorControl_Set.vi"("error in (no error)"=w924, "Output"=-0.1, "Control Mode"=w920, "PhoenixMotorControlDevRef"=w925) -> ("error out"=w922:errorcluster, "PhoenixMotorControlDevRef"=w923:T9)  [unwired: 6 in]
          n257 = Wait (ms)(milliseconds to wait=u32 35) -> ()  [unwired: 1 out]
        }
        n258 = for {
          N: 20 -> [_]
          tunnel: w911 -> [w918] mode=indexing
          tunnel: w910 -> [w917] mode=indexing
          w915 = T13 0 items=["PercentOutput"=0, "Position"=1, "Velocity"=2, "Current"=3, "Follower"=5, "MotionProfile"=6, "MotionMagic"=7, "MotionProfileArc"=10, "Disabled"=15] ("Control Mode")
          n259 = Wait (ms)(milliseconds to wait=u32 50) -> ()  [unwired: 1 out]
          n260 = call <vilib>:"CTRE_Phoenix_MotorControl_Set.vi"("error in (no error)"=w917, "Output"=0.0, "Control Mode"=w915, "PhoenixMotorControlDevRef"=w918) -> ()  [unwired: 6 in, 2 out]
        }
        n261 = Greater?(x=w905, y=2) -> (0:w904:bool)
        n262 = Wait (ms)(milliseconds to wait=u32 20) -> ()  [unwired: 1 out]
      }
      n263 = call <vilib>:"WPI_SwitchRefNum Registry Get.vi"("refnum name"="Orange Limit Switch") -> ("error out"=w871:errorcluster, "SwitchDevRef"=w870:T4)  [unwired: 9 in]
      n264 = call <vilib>:"WPI_SwitchRefNum Registry Get.vi"("refnum name"="Blue Limit Switch") -> ("error out"=w873:errorcluster, "SwitchDevRef"=w872:T4)  [unwired: 9 in]
      n265 = while {
        tunnel: w863 -> [_]
        tunnel: w862 -> [_]
        tunnel: w873 -> [w1131]
        tunnel: w872 -> [w1130]
        tunnel: w871 -> [w1129]
        tunnel: w870 -> [w1128]
        tunnel: w869 -> [w1107]
        tunnel: w868 -> [w1106]
        tunnel: w867 -> [w1102]
        tunnel: w866 -> [w1103]
        tunnel: [w1111] -> w861
        tunnel: [w1110] -> w860
        tunnel: [w1109] -> w859
        tunnel: [w1108] -> w858
        tunnel: [w1107] -> w857
        tunnel: [w1106] -> w856
        tunnel: [w1105] -> w855
        tunnel: [w1104] -> w854
        i -> [w1117]
        stop <- w1116 stop-if-true
        w1101 = T13 0 items=["PercentOutput"=0, "Position"=1, "Velocity"=2, "Current"=3, "Follower"=5, "MotionProfile"=6, "MotionMagic"=7, "MotionProfileArc"=10, "Disabled"=15] ("Control Mode")
        n266 = call <vilib>:"WPI_SwitchGetLimitValue.vi"("error in (no error)"=w1129, "SwitchDevRef"=w1128) -> ("error out"=w1108:errorcluster, "Switch Pressed"=w1127:bool, "SwitchDevRef"=w1109:T4)  [unwired: 7 in]
        "Orange Limit Pressed 3" <- w1127
        n267 = call <vilib>:"WPI_SwitchGetLimitValue.vi"("error in (no error)"=w1131, "SwitchDevRef"=w1130) -> ("error out"=w1110:errorcluster, "Switch Pressed"=w1126:bool, "SwitchDevRef"=w1111:T4)  [unwired: 7 in]
        "Blue Limit Pressed 3" <- w1126
        n268 = call-poly <vilib>:"NT Read Value.vi"("Default Value"=0.0, "Name"="/limelight-drtrain/ty") -> ("Numeric"=w1121:dbl)  [unwired: 8 in, 1 out]
        "Ty 3" <- w1121
        n269 = Greater?(x=w1117, y=5) -> (0:w1116:bool)
        n270 = call "Turret_Aim.vi"("View Button"=FALSE ("Driver Right Thumb"), "Left Trigger"=2.0, "Orange Limit Pressed"=w1126, "Blue Limit Pressed"=w1127, "Right Bumper"=FALSE, "Left Bumper"=FALSE) -> ()  [unwired: 6 in]
        n271 = call "Shooter_Equation.vi"("Right Trigger"=2.0, "Ty"=w1121) -> ()  [unwired: 10 in]
        n272 = Wait (ms)(milliseconds to wait=u32 100) -> ()  [unwired: 1 out]
        n273 = call "Drive_Vi.vi"("Middle Thumb"=FALSE, "Z"=0.0, "Y"=0.15, "X"=0.0) -> ()  [unwired: 8 in]
        n274 = call <vilib>:"CTRE_Phoenix_MotorControl_Set.vi"("error in (no error)"=w1102, "Output"=0.0, "Control Mode"=w1101, "PhoenixMotorControlDevRef"=w1103) -> ("error out"=w1104:errorcluster, "PhoenixMotorControlDevRef"=w1105:T9)  [unwired: 6 in]
      }
      n275 = while {
        tunnel: w860 -> [w1097]
        tunnel: w861 -> [w1096]
        tunnel: w858 -> [w1095]
        tunnel: w857 -> [w1082]
        tunnel: w856 -> [w1081]
        tunnel: w854 -> [w1080]
        tunnel: w855 -> [w1079]
        tunnel: w859 -> [w1070]
        tunnel: [w1069] -> w853
        tunnel: [w1068] -> w852
        tunnel: [w1067] -> w851
        tunnel: [w1066] -> w850
        i -> [w1084]
        stop <- w1083 stop-if-true
        w1077 = T13 0 items=["PercentOutput"=0, "Position"=1, "Velocity"=2, "Current"=3, "Follower"=5, "MotionProfile"=6, "MotionMagic"=7, "MotionProfileArc"=10, "Disabled"=15] ("Control Mode")
        w1078 = T13 0 items=["PercentOutput"=0, "Position"=1, "Velocity"=2, "Current"=3, "Follower"=5, "MotionProfile"=6, "MotionMagic"=7, "MotionProfileArc"=10, "Disabled"=15] ("Control Mode")
        # "40"
        n276 = call <vilib>:"WPI_SwitchGetLimitValue.vi"("error in (no error)"=w1095, "SwitchDevRef"=w1070) -> ("Switch Pressed"=w1094:bool)  [unwired: 7 in, 2 out]
        "Orange Limit Pressed 4" <- w1094
        n277 = call <vilib>:"WPI_SwitchGetLimitValue.vi"("error in (no error)"=w1097, "SwitchDevRef"=w1096) -> ("Switch Pressed"=w1093:bool)  [unwired: 7 in, 2 out]
        "Blue Limit Pressed 4" <- w1093
        n278 = call-poly <vilib>:"NT Read Value.vi"("Default Value"=0.0, "Name"="/limelight-drtrain/ty") -> ("Numeric"=w1088:dbl)  [unwired: 8 in, 1 out]
        "Ty 4" <- w1088
        n279 = Greater?(x=w1084, y=20) -> (0:w1083:bool)
        n280 = call "Turret_Aim.vi"("View Button"=FALSE ("Driver Right Thumb"), "Left Trigger"=2.0, "Orange Limit Pressed"=w1093, "Blue Limit Pressed"=w1094, "Right Bumper"=FALSE, "Left Bumper"=FALSE) -> ()  [unwired: 6 in]
        n281 = call "Shooter_Equation.vi"("Right Trigger"=2.0, "Ty"=w1088) -> ()  [unwired: 10 in]
        n282 = Wait (ms)(milliseconds to wait=u32 100) -> ()  [unwired: 1 out]
        n283 = call "Drive_Vi.vi"("Middle Thumb"=FALSE, "Z"=0.0, "Y"=0.15, "X"=0.0) -> ()  [unwired: 8 in]
        n284 = call <vilib>:"CTRE_Phoenix_MotorControl_Set.vi"("error in (no error)"=w1080, "Output"=0.35, "Control Mode"=w1077, "PhoenixMotorControlDevRef"=w1079) -> ("error out"=w1069:errorcluster, "PhoenixMotorControlDevRef"=w1068:T9)  [unwired: 6 in]
        n285 = call <vilib>:"CTRE_Phoenix_MotorControl_Set.vi"("error in (no error)"=w1082, "Output"=-0.35, "Control Mode"=w1078, "PhoenixMotorControlDevRef"=w1081) -> ("error out"=w1066:errorcluster, "PhoenixMotorControlDevRef"=w1067:T9)  [unwired: 6 in]
      }
      n286 = while {
        tunnel: w853 -> [w1061]
        tunnel: w852 -> [w1060]
        tunnel: w851 -> [w1059]
        tunnel: w850 -> [w1058]
        tunnel: [w1049] -> w830
        tunnel: [w1048] -> w828
        tunnel: [w1047] -> w826
        tunnel: [w1046] -> w824
        i -> [w1056]
        stop <- w1055 stop-if-true
        w1064 = T13 0 items=["PercentOutput"=0, "Position"=1, "Velocity"=2, "Current"=3, "Follower"=5, "MotionProfile"=6, "MotionMagic"=7, "MotionProfileArc"=10, "Disabled"=15] ("Control Mode")
        w1065 = T13 0 items=["PercentOutput"=0, "Position"=1, "Velocity"=2, "Current"=3, "Follower"=5, "MotionProfile"=6, "MotionMagic"=7, "MotionProfileArc"=10, "Disabled"=15] ("Control Mode")
        n287 = call <vilib>:"CTRE_Phoenix_MotorControl_Set.vi"("error in (no error)"=w1061, "Output"=0.0, "Control Mode"=w1064, "PhoenixMotorControlDevRef"=w1060) -> ("error out"=w1048:errorcluster, "PhoenixMotorControlDevRef"=w1049:T9)  [unwired: 6 in]
        n288 = call <vilib>:"CTRE_Phoenix_MotorControl_Set.vi"("error in (no error)"=w1058, "Output"=0.0, "Control Mode"=w1065, "PhoenixMotorControlDevRef"=w1059) -> ("error out"=w1046:errorcluster, "PhoenixMotorControlDevRef"=w1047:T9)  [unwired: 6 in]
        n289 = call "Drive_Vi.vi"("Middle Thumb"=FALSE, "Z"=-0.35, "Y"=0.0, "X"=0.0) -> ()  [unwired: 8 in]
        n290 = Greater?(x=w1056, y=5) -> (0:w1055:bool)
        n291 = Wait (ms)(milliseconds to wait=u32 100) -> ()  [unwired: 1 out]
        n292 = call-poly <vilib>:"NT Read Value.vi"("Default Value"=0.0, "Name"="/limelight-drtrain/ty") -> ("Numeric"=w1051:dbl)  [unwired: 8 in, 1 out]
        "Ty 9" <- w1051
        n293 = call "Shooter_Equation.vi"("Right Trigger"=0.0, "Ty"=w1051) -> ()  [unwired: 10 in]
      }
      n294 = while {
        tunnel: [w895] -> w829
        tunnel: w830 -> [w895]
        tunnel: [w894] -> w827
        tunnel: w828 -> [w894]
        tunnel: [w893] -> w825
        tunnel: w826 -> [w893]
        tunnel: [w892] -> w823
        tunnel: w824 -> [w892]
        i -> [w901]
        stop <- w902 stop-if-true
        n295 = Wait (ms)(milliseconds to wait=u32 20) -> ()  [unwired: 1 out]
        n296 = Greater?(x=w901, y=5) -> (0:w902:bool)
        n297 = call "Drive_Vi.vi"("Middle Thumb"=TRUE, "Z"=0.0, "Y"=0.0, "X"=0.0) -> ()  [unwired: 8 in]
      }
      n298 = while {
        tunnel: w829 -> [w1025]
        tunnel: w827 -> [w1024]
        tunnel: w825 -> [w1023]
        tunnel: w823 -> [w1022]
        tunnel: [w1021] -> w849
        tunnel: [w1020] -> w848
        tunnel: [w1019] -> w847
        tunnel: [w1018] -> w846
        i -> [w1036]
        stop <- w1035 stop-if-true
        w1040 = T13 0 items=["PercentOutput"=0, "Position"=1, "Velocity"=2, "Current"=3, "Follower"=5, "MotionProfile"=6, "MotionMagic"=7, "MotionProfileArc"=10, "Disabled"=15] ("Control Mode")
        w1041 = T13 0 items=["PercentOutput"=0, "Position"=1, "Velocity"=2, "Current"=3, "Follower"=5, "MotionProfile"=6, "MotionMagic"=7, "MotionProfileArc"=10, "Disabled"=15] ("Control Mode")
        # "-0.186"
        # "-0.944"
        # ".135"
        n299 = call "Drive_Vi.vi"("Middle Thumb"=FALSE, "Z"=0.0, "Y"=-0.8, "X"=0.0) -> ()  [unwired: 8 in]
        n300 = call <vilib>:"CTRE_Phoenix_MotorControl_Set.vi"("error in (no error)"=w1024, "Output"=0.0, "Control Mode"=w1040, "PhoenixMotorControlDevRef"=w1025) -> ("error out"=w1020:errorcluster, "PhoenixMotorControlDevRef"=w1021:T9)  [unwired: 6 in]
        n301 = call <vilib>:"CTRE_Phoenix_MotorControl_Set.vi"("error in (no error)"=w1022, "Output"=0.0, "Control Mode"=w1041, "PhoenixMotorControlDevRef"=w1023) -> ("error out"=w1018:errorcluster, "PhoenixMotorControlDevRef"=w1019:T9)  [unwired: 6 in]
        n302 = Greater?(x=w1036, y=8) -> (0:w1035:bool)
        n303 = Wait (ms)(milliseconds to wait=u32 100) -> ()  [unwired: 1 out]
        n304 = call-poly <vilib>:"NT Read Value.vi"("Default Value"=0.0, "Name"="/limelight-drtrain/ty") -> ("Numeric"=w1027:dbl)  [unwired: 8 in, 1 out]
        "Ty 10" <- w1027
        n305 = call "Shooter_Equation.vi"("Right Trigger"=0.0, "Ty"=w1027) -> ()  [unwired: 10 in]
      }
      n306 = while {
        tunnel: w849 -> [w1009]
        tunnel: w848 -> [w1008]
        tunnel: w847 -> [w1007]
        tunnel: w846 -> [w1006]
        tunnel: [w1001] -> w845
        tunnel: [w1000] -> w844
        tunnel: [w999] -> w843
        tunnel: [w998] -> w842
        i -> [w1003]
        stop <- w1002 stop-if-true
        w1016 = T13 0 items=["PercentOutput"=0, "Position"=1, "Velocity"=2, "Current"=3, "Follower"=5, "MotionProfile"=6, "MotionMagic"=7, "MotionProfileArc"=10, "Disabled"=15] ("Control Mode")
        w1017 = T13 0 items=["PercentOutput"=0, "Position"=1, "Velocity"=2, "Current"=3, "Follower"=5, "MotionProfile"=6, "MotionMagic"=7, "MotionProfileArc"=10, "Disabled"=15] ("Control Mode")
        # "-0.186"
        # "-0.944"
        # ".135"
        n307 = call <vilib>:"CTRE_Phoenix_MotorControl_Set.vi"("error in (no error)"=w1008, "Output"=0.0, "Control Mode"=w1016, "PhoenixMotorControlDevRef"=w1009) -> ("error out"=w1000:errorcluster, "PhoenixMotorControlDevRef"=w1001:T9)  [unwired: 6 in]
        n308 = call <vilib>:"CTRE_Phoenix_MotorControl_Set.vi"("error in (no error)"=w1006, "Output"=0.0, "Control Mode"=w1017, "PhoenixMotorControlDevRef"=w1007) -> ("error out"=w998:errorcluster, "PhoenixMotorControlDevRef"=w999:T9)  [unwired: 6 in]
        n309 = call "Drive_Vi.vi"("Middle Thumb"=FALSE, "Z"=0.0, "Y"=0.0, "X"=0.0) -> ()  [unwired: 8 in]
        n310 = Greater?(x=w1003, y=5) -> (0:w1002:bool)
        n311 = call-poly <vilib>:"NT Read Value.vi"("Default Value"=0.0, "Name"="/limelight-drtrain/ty") -> ("Numeric"=w1011:dbl)  [unwired: 8 in, 1 out]
        "Ty 11" <- w1011
        n312 = Wait (ms)(milliseconds to wait=u32 100) -> ()  [unwired: 1 out]
        n313 = call "Shooter_Equation.vi"("Right Trigger"=0.0, "Ty"=w1011) -> ()  [unwired: 10 in]
      }
      n314 = while {
        tunnel: w845 -> [w981]
        tunnel: w844 -> [w980]
        tunnel: w843 -> [w979]
        tunnel: w842 -> [w978]
        tunnel: [w973] -> w841
        tunnel: [w972] -> w840
        tunnel: [w971] -> w839
        tunnel: [w970] -> w838
        i -> [w975]
        stop <- w974 stop-if-true
        w992 = T13 0 items=["PercentOutput"=0, "Position"=1, "Velocity"=2, "Current"=3, "Follower"=5, "MotionProfile"=6, "MotionMagic"=7, "MotionProfileArc"=10, "Disabled"=15] ("Control Mode")
        w993 = T13 0 items=["PercentOutput"=0, "Position"=1, "Velocity"=2, "Current"=3, "Follower"=5, "MotionProfile"=6, "MotionMagic"=7, "MotionProfileArc"=10, "Disabled"=15] ("Control Mode")
        # "-0.186"
        # "-0.944"
        # ".135"
        n315 = call "Drive_Vi.vi"("Middle Thumb"=FALSE, "Z"=0.0, "Y"=0.0, "X"=0.0) -> ()  [unwired: 8 in]
        n316 = call <vilib>:"CTRE_Phoenix_MotorControl_Set.vi"("error in (no error)"=w980, "Output"=0.75, "Control Mode"=w992, "PhoenixMotorControlDevRef"=w981) -> ("error out"=w972:errorcluster, "PhoenixMotorControlDevRef"=w973:T9)  [unwired: 6 in]
        n317 = call <vilib>:"CTRE_Phoenix_MotorControl_Set.vi"("error in (no error)"=w978, "Output"=-0.1, "Control Mode"=w993, "PhoenixMotorControlDevRef"=w979) -> ("error out"=w970:errorcluster, "PhoenixMotorControlDevRef"=w971:T9)  [unwired: 6 in]
        n318 = Greater?(x=w975, y=20) -> (0:w974:bool)
        n319 = Wait (ms)(milliseconds to wait=u32 100) -> ()  [unwired: 1 out]
        n320 = call-poly <vilib>:"NT Read Value.vi"("Default Value"=0.0, "Name"="/limelight-drtrain/ty") -> ("Numeric"=w983:dbl)  [unwired: 8 in, 1 out]
        "Ty 12" <- w983
        n321 = call "Shooter_Equation.vi"("Right Trigger"=0.0, "Ty"=w983) -> ()  [unwired: 10 in]
      }
      n322 = while {
        tunnel: w841 -> [w957]
        tunnel: [w950] -> _
        tunnel: w839 -> [w956]
        tunnel: w838 -> [w955]
        tunnel: w840 -> [w950]
        tunnel: [w949] -> w837
        tunnel: [w948] -> w836
        tunnel: [w947] -> w835
        tunnel: [w946] -> w834
        i -> [w952]
        stop <- w951 stop-if-true
        w968 = T13 0 items=["PercentOutput"=0, "Position"=1, "Velocity"=2, "Current"=3, "Follower"=5, "MotionProfile"=6, "MotionMagic"=7, "MotionProfileArc"=10, "Disabled"=15] ("Control Mode")
        w969 = T13 0 items=["PercentOutput"=0, "Position"=1, "Velocity"=2, "Current"=3, "Follower"=5, "MotionProfile"=6, "MotionMagic"=7, "MotionProfileArc"=10, "Disabled"=15] ("Control Mode")
        # "-0.186"
        # "-0.944"
        # ".135"
        n323 = call "Drive_Vi.vi"("Middle Thumb"=FALSE, "Z"=0.0, "Y"=0.0, "X"=0.0) -> ()  [unwired: 8 in]
        n324 = call <vilib>:"CTRE_Phoenix_MotorControl_Set.vi"("error in (no error)"=w950, "Output"=0.0, "Control Mode"=w968, "PhoenixMotorControlDevRef"=w957) -> ("error out"=w946:errorcluster, "PhoenixMotorControlDevRef"=w947:T9)  [unwired: 6 in]
        n325 = call <vilib>:"CTRE_Phoenix_MotorControl_Set.vi"("error in (no error)"=w955, "Output"=0.0, "Control Mode"=w969, "PhoenixMotorControlDevRef"=w956) -> ("error out"=w949:errorcluster, "PhoenixMotorControlDevRef"=w948:T9)  [unwired: 6 in]
        n326 = Greater?(x=w952, y=10) -> (0:w951:bool)
        n327 = Wait (ms)(milliseconds to wait=u32 100) -> ()  [unwired: 1 out]
        n328 = call-poly <vilib>:"NT Read Value.vi"("Default Value"=0.0, "Name"="/limelight-drtrain/ty") -> ("Numeric"=w959:dbl)  [unwired: 8 in, 1 out]
        "Ty 13" <- w959
        n329 = call "Shooter_Equation.vi"("Right Trigger"=0.0, "Ty"=w959) -> ()  [unwired: 10 in]
      }
      n330 = while {
        tunnel: w835 -> [w933]
        tunnel: [w926] -> _
        tunnel: w836 -> [w932]
        tunnel: w837 -> [w931]
        tunnel: w834 -> [w926]
        i -> [w928]
        stop <- w927 stop-if-true
        w944 = T13 0 items=["PercentOutput"=0, "Position"=1, "Velocity"=2, "Current"=3, "Follower"=5, "MotionProfile"=6, "MotionMagic"=7, "MotionProfileArc"=10, "Disabled"=15] ("Control Mode")
        w945 = T13 0 items=["PercentOutput"=0, "Position"=1, "Velocity"=2, "Current"=3, "Follower"=5, "MotionProfile"=6, "MotionMagic"=7, "MotionProfileArc"=10, "Disabled"=15] ("Control Mode")
        # "-0.186"
        # "-0.944"
        # ".135"
        n331 = call "Drive_Vi.vi"("Middle Thumb"=FALSE, "Z"=0.0, "Y"=0.0, "X"=0.0) -> ()  [unwired: 8 in]
        n332 = call <vilib>:"CTRE_Phoenix_MotorControl_Set.vi"("error in (no error)"=w926, "Output"=0.0, "Control Mode"=w944, "PhoenixMotorControlDevRef"=w933) -> ()  [unwired: 6 in, 2 out]
        n333 = call <vilib>:"CTRE_Phoenix_MotorControl_Set.vi"("error in (no error)"=w931, "Output"=0.0, "Control Mode"=w945, "PhoenixMotorControlDevRef"=w932) -> ()  [unwired: 6 in, 2 out]
        n334 = Greater?(x=w928, y=20) -> (0:w927:bool)
        n335 = Wait (ms)(milliseconds to wait=u32 100) -> ()  [unwired: 1 out]
        n336 = call-poly <vilib>:"NT Read Value.vi"("Default Value"=0.0, "Name"="/limelight-drtrain/ty") -> ("Numeric"=w935:dbl)  [unwired: 8 in, 1 out]
        "Ty 14" <- w935
        n337 = call "Shooter_Equation.vi"("Right Trigger"=0.0, "Ty"=w935) -> ()  [unwired: 10 in]
      }
    }
    frame "4 Ball Pos 3" {
      # "Pigeon Set"
      n338 = while {
        i -> [w1624]
        stop <- w1625 stop-if-true
        n339 = Wait (ms)(milliseconds to wait=u32 20) -> ()  [unwired: 1 out]
        n340 = Greater?(x=w1624, y=2) -> (0:w1625:bool)
        n341 = call "Drive_Vi.vi"("Middle Thumb"=TRUE, "Z"=0.0, "Y"=0.0, "X"=0.0) -> ()  [unwired: 8 in]
      }
      n342 = call <vilib>:"WPI_SwitchRefNum Registry Get.vi"("refnum name"="Intake Sensor") -> ("error out"=w1277:errorcluster, "SwitchDevRef"=w1276:T4)  [unwired: 9 in]
      n343 = call <vilib>:"CTRE_Phoenix_MotorControl_RefNumRegistryGet.vi"("refnum name"="Intake") -> ("error out"=w1271:errorcluster, "PhoenixMotorControlDevRef"=w1270:T9)  [unwired: 9 in]
      n344 = call <vilib>:"CTRE_Phoenix_MotorControl_RefNumRegistryGet.vi"("refnum name"="Reject") -> ("error out"=w1273:errorcluster, "PhoenixMotorControlDevRef"=w1272:T9)  [unwired: 9 in]
      n345 = call "Limit_Switches.vi"() -> ()  [unwired: 10 in, 2 out]
      n346 = call <vilib>:"CTRE_Phoenix_MotorControl_RefNumRegistryGet.vi"("refnum name"="Elevate") -> ("error out"=w1275:errorcluster, "PhoenixMotorControlDevRef"=w1274:T9)  [unwired: 9 in]
      n347 = call <vilib>:"WPI_SwitchRefNum Registry Get.vi"("refnum name"="Elevate Sensor") -> ("error out"=w1279:errorcluster, "SwitchDevRef"=w1278:T4)  [unwired: 9 in]
      n348 = call <vilib>:"CTRE_Phoenix_MotorControl_RefNumRegistryGet.vi"("refnum name"="Shoot") -> ("error out"=w1259:errorcluster, "PhoenixMotorControlDevRef"=w1258:T9)  [unwired: 9 in]
      n349 = call <vilib>:"CTRE_Phoenix_MotorControl_RefNumRegistryGet.vi"("refnum name"="Intake Actuate") -> ("error out"=w1229:errorcluster, "PhoenixMotorControlDevRef"=w1230:T9)  [unwired: 9 in]
      n350 = while {
        tunnel: w1279 -> [w1583]
        tunnel: w1278 -> [w1582]
        tunnel: w1277 -> [w1581]
        tunnel: w1276 -> [w1580]
        tunnel: w1275 -> [w1577]
        tunnel: w1274 -> [w1576]
        tunnel: w1273 -> [w1575]
        tunnel: w1272 -> [w1574]
        tunnel: w1271 -> [w1573]
        tunnel: w1270 -> [w1572]
        tunnel: [w1561] -> w1263
        tunnel: [w1560] -> w1262
        tunnel: [w1559] -> w1261
        tunnel: [w1558] -> w1260
        tunnel: w1259 -> [w1557]
        tunnel: w1258 -> [w1556]
        tunnel: [w1553] -> w1257
        tunnel: [w1552] -> w1256
        i -> [w1586]
        stop <- w1587 stop-if-true
        w1555 = T13 0 items=["PercentOutput"=0, "Position"=1, "Velocity"=2, "Current"=3, "Follower"=5, "MotionProfile"=6, "MotionMagic"=7, "MotionProfileArc"=10, "Disabled"=15] ("Control Mode")
        w1566 = T13 0 items=["PercentOutput"=0, "Position"=1, "Velocity"=2, "Current"=3, "Follower"=5, "MotionProfile"=6, "MotionMagic"=7, "MotionProfileArc"=10, "Disabled"=15] ("Control Mode")
        w1567 = T13 0 items=["PercentOutput"=0, "Position"=1, "Velocity"=2, "Current"=3, "Follower"=5, "MotionProfile"=6, "MotionMagic"=7, "MotionProfileArc"=10, "Disabled"=15] ("Control Mode")
        w1568 = T13 0 items=["PercentOutput"=0, "Position"=1, "Velocity"=2, "Current"=3, "Follower"=5, "MotionProfile"=6, "MotionMagic"=7, "MotionProfileArc"=10, "Disabled"=15] ("Control Mode")
        n351 = call <vilib>:"WPI_SwitchGetLimitValue.vi"("error in (no error)"=w1581, "SwitchDevRef"=w1580) -> ("Switch Pressed"=w1584:bool)  [unwired: 7 in, 2 out]
        n352 = call <vilib>:"WPI_SwitchGetLimitValue.vi"("error in (no error)"=w1583, "SwitchDevRef"=w1582) -> ("Switch Pressed"=w1585:bool)  [unwired: 7 in, 2 out]
        n353 = Greater?(x=w1586, y=20) -> (0:w1587:bool)
        n354 = Not(x=w1584) -> (.not. x?=w1571:bool)
        "Intake 5" <- w1571
        n355 = Not(x=w1585) -> (.not. x?=w1579:bool)
        "Elevate 5" <- w1579
        n356 = Wait (ms)(milliseconds to wait=u32 100) -> ()  [unwired: 1 out]
        n357 = case shown="True" w1579 {
          tunnel: [0.75 ("Output") w1604] -> w1578
          tunnel: w1571 -> [_ w1601]
          tunnel: [0.75 ("Output") w1603] -> w1570
          tunnel: [-0.1 ("Output") w1602] -> w1569
          tunnel: [FALSE ("Middle Thumb") w1600] -> w1565
          tunnel: [0.0 ("Z") w1599] -> w1564
          tunnel: [0.0 ("Y") w1598] -> w1563
          tunnel: [0.0 ("X") w1597] -> w1562
          frame False {
            (unwired) WPI_SolenoidValue."Reverse" ("Value")
          }
          frame True {
            n358 = case shown="True" w1601 {
              tunnel: [0.75 ("Output") 0.0 ("Output")] -> w1604
              tunnel: [0.0 ("Output") 0.0 ("Output")] -> w1603
              tunnel: [0.0 ("Output") 0.0 ("Output")] -> w1602
              tunnel: [FALSE ("Middle Thumb") FALSE ("Middle Thumb")] -> w1600
              tunnel: [0.0 ("Z") 0.0 ("Z")] -> w1599
              tunnel: [-0.3 ("Y") 0.0 ("Y")] -> w1598
              tunnel: [0.0 ("X") 0.0 ("X")] -> w1597
              frame False {
              }
              frame True {
              }
            }
          }
        }
        n359 = call <vilib>:"CTRE_Phoenix_MotorControl_Set.vi"("error in (no error)"=w1573, "Output"=w1578, "Control Mode"=w1566, "PhoenixMotorControlDevRef"=w1572) -> ("error out"=w1559:errorcluster, "PhoenixMotorControlDevRef"=w1558:T9)  [unwired: 6 in]
        n360 = call <vilib>:"CTRE_Phoenix_MotorControl_Set.vi"("error in (no error)"=w1575, "Output"=w1570, "Control Mode"=w1567, "PhoenixMotorControlDevRef"=w1574) -> ()  [unwired: 6 in, 2 out]
        n361 = call <vilib>:"CTRE_Phoenix_MotorControl_Set.vi"("error in (no error)"=w1577, "Output"=w1569, "Control Mode"=w1568, "PhoenixMotorControlDevRef"=w1576) -> ("error out"=w1561:errorcluster, "PhoenixMotorControlDevRef"=w1560:T9)  [unwired: 6 in]
        n362 = call <vilib>:"CTRE_Phoenix_MotorControl_Set.vi"("error in (no error)"=w1557, "Output"=-0.55, "Control Mode"=w1555, "PhoenixMotorControlDevRef"=w1556) -> ("error out"=w1553:errorcluster, "PhoenixMotorControlDevRef"=w1552:T9)  [unwired: 6 in]
        n363 = call "Drive_Vi.vi"("Middle Thumb"=w1565, "Z"=w1564, "Y"=w1563, "X"=w1562) -> ()  [unwired: 8 in]
      }
      n364 = while {
        tunnel: w1230 -> [w1319]
        tunnel: w1229 -> [w1318]
        i -> [w1311]
        stop <- w1310 stop-if-true
        n365 = for {
          N: 20 -> [_]
          tunnel: w1319 -> [w1331]
          tunnel: w1318 -> [w1330]
          tunnel: [w1329] -> w1317 mode=indexing
          tunnel: [w1328] -> w1316 mode=indexing
          w1326 = T13 0 items=["PercentOutput"=0, "Position"=1, "Velocity"=2, "Current"=3, "Follower"=5, "MotionProfile"=6, "MotionMagic"=7, "MotionProfileArc"=10, "Disabled"=15] ("Control Mode")
          n366 = call <vilib>:"CTRE_Phoenix_MotorControl_Set.vi"("error in (no error)"=w1330, "Output"=-0.1, "Control Mode"=w1326, "PhoenixMotorControlDevRef"=w1331) -> ("error out"=w1328:errorcluster, "PhoenixMotorControlDevRef"=w1329:T9)  [unwired: 6 in]
          n367 = Wait (ms)(milliseconds to wait=u32 35) -> ()  [unwired: 1 out]
        }
        n368 = for {
          N: 20 -> [_]
          tunnel: w1317 -> [w1324] mode=indexing
          tunnel: w1316 -> [w1323] mode=indexing
          w1321 = T13 0 items=["PercentOutput"=0, "Position"=1, "Velocity"=2, "Current"=3, "Follower"=5, "MotionProfile"=6, "MotionMagic"=7, "MotionProfileArc"=10, "Disabled"=15] ("Control Mode")
          n369 = Wait (ms)(milliseconds to wait=u32 50) -> ()  [unwired: 1 out]
          n370 = call <vilib>:"CTRE_Phoenix_MotorControl_Set.vi"("error in (no error)"=w1323, "Output"=0.0, "Control Mode"=w1321, "PhoenixMotorControlDevRef"=w1324) -> ()  [unwired: 6 in, 2 out]
        }
        n371 = Greater?(x=w1311, y=2) -> (0:w1310:bool)
        n372 = Wait (ms)(milliseconds to wait=u32 20) -> ()  [unwired: 1 out]
      }
      n373 = call <vilib>:"WPI_SwitchRefNum Registry Get.vi"("refnum name"="Orange Limit Switch") -> ("error out"=w1265:errorcluster, "SwitchDevRef"=w1264:T4)  [unwired: 9 in]
      n374 = call <vilib>:"WPI_SwitchRefNum Registry Get.vi"("refnum name"="Blue Limit Switch") -> ("error out"=w1267:errorcluster, "SwitchDevRef"=w1266:T4)  [unwired: 9 in]
      n375 = while {
        tunnel: w1257 -> [_]
        tunnel: w1256 -> [_]
        tunnel: w1267 -> [w1549]
        tunnel: w1266 -> [w1548]
        tunnel: w1265 -> [w1547]
        tunnel: w1264 -> [w1546]
        tunnel: w1263 -> [w1525]
        tunnel: w1262 -> [w1524]
        tunnel: w1261 -> [w1520]
        tunnel: w1260 -> [w1521]
        tunnel: [w1529] -> w1255
        tunnel: [w1528] -> w1254
        tunnel: [w1527] -> w1253
        tunnel: [w1526] -> w1252
        tunnel: [w1525] -> w1251
        tunnel: [w1524] -> w1250
        tunnel: [w1523] -> w1249
        tunnel: [w1522] -> w1248
        i -> [w1535]
        stop <- w1534 stop-if-true
        w1519 = T13 0 items=["PercentOutput"=0, "Position"=1, "Velocity"=2, "Current"=3, "Follower"=5, "MotionProfile"=6, "MotionMagic"=7, "MotionProfileArc"=10, "Disabled"=15] ("Control Mode")
        n376 = call <vilib>:"WPI_SwitchGetLimitValue.vi"("error in (no error)"=w1547, "SwitchDevRef"=w1546) -> ("error out"=w1526:errorcluster, "Switch Pressed"=w1545:bool, "SwitchDevRef"=w1527:T4)  [unwired: 7 in]
        "Orange Limit Pressed 9" <- w1545
        n377 = call <vilib>:"WPI_SwitchGetLimitValue.vi"("error in (no error)"=w1549, "SwitchDevRef"=w1548) -> ("error out"=w1528:errorcluster, "Switch Pressed"=w1544:bool, "SwitchDevRef"=w1529:T4)  [unwired: 7 in]
        "Blue Limit Pressed 9" <- w1544
        n378 = call-poly <vilib>:"NT Read Value.vi"("Default Value"=0.0, "Name"="/limelight-drtrain/ty") -> ("Numeric"=w1539:dbl)  [unwired: 8 in, 1 out]
        "Ty 15" <- w1539
        n379 = Greater?(x=w1535, y=5) -> (0:w1534:bool)
        n380 = call "Turret_Aim.vi"("View Button"=FALSE ("Driver Right Thumb"), "Left Trigger"=2.0, "Orange Limit Pressed"=w1544, "Blue Limit Pressed"=w1545, "Right Bumper"=FALSE, "Left Bumper"=FALSE) -> ()  [unwired: 6 in]
        n381 = call "Shooter_Equation.vi"("Right Trigger"=2.0, "Ty"=w1539) -> ()  [unwired: 10 in]
        n382 = Wait (ms)(milliseconds to wait=u32 100) -> ()  [unwired: 1 out]
        n383 = call "Drive_Vi.vi"("Middle Thumb"=FALSE, "Z"=0.0, "Y"=0.15, "X"=0.0) -> ()  [unwired: 8 in]
        n384 = call <vilib>:"CTRE_Phoenix_MotorControl_Set.vi"("error in (no error)"=w1520, "Output"=0.0, "Control Mode"=w1519, "PhoenixMotorControlDevRef"=w1521) -> ("error out"=w1522:errorcluster, "PhoenixMotorControlDevRef"=w1523:T9)  [unwired: 6 in]
      }
      n385 = while {
        tunnel: w1254 -> [w1515]
        tunnel: w1255 -> [w1514]
        tunnel: w1252 -> [w1513]
        tunnel: w1251 -> [w1502]
        tunnel: w1250 -> [w1501]
        tunnel: w1248 -> [w1500]
        tunnel: w1249 -> [w1499]
        tunnel: w1253 -> [w1490]
        tunnel: [w1489] -> w1247
        tunnel: [w1488] -> w1246
        tunnel: [w1487] -> w1245
        tunnel: [w1486] -> w1244
        tunnel: [w1485] -> w1212
        tunnel: [w1484] -> w1211
        i -> [w1504]
        stop <- w1503 stop-if-true
        w1497 = T13 0 items=["PercentOutput"=0, "Position"=1, "Velocity"=2, "Current"=3, "Follower"=5, "MotionProfile"=6, "MotionMagic"=7, "MotionProfileArc"=10, "Disabled"=15] ("Control Mode")
        w1498 = T13 0 items=["PercentOutput"=0, "Position"=1, "Velocity"=2, "Current"=3, "Follower"=5, "MotionProfile"=6, "MotionMagic"=7, "MotionProfileArc"=10, "Disabled"=15] ("Control Mode")
        # "40"
        n386 = call <vilib>:"WPI_SwitchGetLimitValue.vi"("error in (no error)"=w1513, "SwitchDevRef"=w1490) -> ("Switch Pressed"=w1485:bool)  [unwired: 7 in, 2 out]
        "Orange Limit Pressed 10" <- w1485
        n387 = call <vilib>:"WPI_SwitchGetLimitValue.vi"("error in (no error)"=w1515, "SwitchDevRef"=w1514) -> ("Switch Pressed"=w1484:bool)  [unwired: 7 in, 2 out]
        "Blue Limit Pressed 10" <- w1484
        n388 = call-poly <vilib>:"NT Read Value.vi"("Default Value"=0.0, "Name"="/limelight-drtrain/ty") -> ("Numeric"=w1508:dbl)  [unwired: 8 in, 1 out]
        "Ty 16" <- w1508
        n389 = Greater?(x=w1504, y=20) -> (0:w1503:bool)
        n390 = call "Turret_Aim.vi"("View Button"=FALSE ("Driver Right Thumb"), "Left Trigger"=2.0, "Orange Limit Pressed"=w1484, "Blue Limit Pressed"=w1485, "Right Bumper"=FALSE, "Left Bumper"=FALSE) -> ()  [unwired: 6 in]
        n391 = call "Shooter_Equation.vi"("Right Trigger"=2.0, "Ty"=w1508) -> ()  [unwired: 10 in]
        n392 = Wait (ms)(milliseconds to wait=u32 100) -> ()  [unwired: 1 out]
        n393 = call "Drive_Vi.vi"("Middle Thumb"=FALSE, "Z"=0.0, "Y"=0.15, "X"=0.0) -> ()  [unwired: 8 in]
        n394 = call <vilib>:"CTRE_Phoenix_MotorControl_Set.vi"("error in (no error)"=w1500, "Output"=0.35, "Control Mode"=w1497, "PhoenixMotorControlDevRef"=w1499) -> ("error out"=w1489:errorcluster, "PhoenixMotorControlDevRef"=w1488:T9)  [unwired: 6 in]
        n395 = call <vilib>:"CTRE_Phoenix_MotorControl_Set.vi"("error in (no error)"=w1502, "Output"=-0.35, "Control Mode"=w1498, "PhoenixMotorControlDevRef"=w1501) -> ("error out"=w1486:errorcluster, "PhoenixMotorControlDevRef"=w1487:T9)  [unwired: 6 in]
      }
      n396 = while {
        tunnel: w1247 -> [w1479]
        tunnel: w1246 -> [w1478]
        tunnel: w1245 -> [w1477]
        tunnel: w1244 -> [w1476]
        tunnel: [w1467] -> w1228
        tunnel: [w1466] -> w1226
        tunnel: [w1465] -> w1224
        tunnel: [w1464] -> w1222
        i -> [w1474]
        stop <- w1473 stop-if-true
        w1482 = T13 0 items=["PercentOutput"=0, "Position"=1, "Velocity"=2, "Current"=3, "Follower"=5, "MotionProfile"=6, "MotionMagic"=7, "MotionProfileArc"=10, "Disabled"=15] ("Control Mode")
        w1483 = T13 0 items=["PercentOutput"=0, "Position"=1, "Velocity"=2, "Current"=3, "Follower"=5, "MotionProfile"=6, "MotionMagic"=7, "MotionProfileArc"=10, "Disabled"=15] ("Control Mode")
        n397 = call <vilib>:"CTRE_Phoenix_MotorControl_Set.vi"("error in (no error)"=w1479, "Output"=0.0, "Control Mode"=w1482, "PhoenixMotorControlDevRef"=w1478) -> ("error out"=w1466:errorcluster, "PhoenixMotorControlDevRef"=w1467:T9)  [unwired: 6 in]
        n398 = call <vilib>:"CTRE_Phoenix_MotorControl_Set.vi"("error in (no error)"=w1476, "Output"=0.0, "Control Mode"=w1483, "PhoenixMotorControlDevRef"=w1477) -> ("error out"=w1464:errorcluster, "PhoenixMotorControlDevRef"=w1465:T9)  [unwired: 6 in]
        n399 = call "Drive_Vi.vi"("Middle Thumb"=FALSE, "Z"=0.22, "Y"=0.0, "X"=0.0) -> ()  [unwired: 8 in]
        n400 = Greater?(x=w1474, y=4) -> (0:w1473:bool)
        n401 = Wait (ms)(milliseconds to wait=u32 100) -> ()  [unwired: 1 out]
        n402 = call-poly <vilib>:"NT Read Value.vi"("Default Value"=0.0, "Name"="/limelight-drtrain/ty") -> ("Numeric"=w1469:dbl)  [unwired: 8 in, 1 out]
        "Ty 17" <- w1469
        n403 = call "Shooter_Equation.vi"("Right Trigger"=0.0, "Ty"=w1469) -> ()  [unwired: 10 in]
      }
      n404 = while {
        tunnel: [w1301] -> w1227
        tunnel: w1228 -> [w1301]
        tunnel: [w1300] -> w1225
        tunnel: w1226 -> [w1300]
        tunnel: [w1299] -> w1223
        tunnel: w1224 -> [w1299]
        tunnel: [w1298] -> w1221
        tunnel: w1222 -> [w1298]
        i -> [w1307]
        stop <- w1308 stop-if-true
        n405 = Wait (ms)(milliseconds to wait=u32 20) -> ()  [unwired: 1 out]
        n406 = Greater?(x=w1307, y=5) -> (0:w1308:bool)
        n407 = call "Drive_Vi.vi"("Middle Thumb"=TRUE, "Z"=0.0, "Y"=0.0, "X"=0.0) -> ()  [unwired: 8 in]
      }
      n408 = while {
        tunnel: w1227 -> [w1443]
        tunnel: w1225 -> [w1442]
        tunnel: w1223 -> [w1441]
        tunnel: w1221 -> [w1440]
        tunnel: [w1439] -> w1243
        tunnel: [w1438] -> w1242
        tunnel: [w1437] -> w1241
        tunnel: [w1436] -> w1240
        i -> [w1454]
        stop <- w1453 stop-if-true
        w1458 = T13 0 items=["PercentOutput"=0, "Position"=1, "Velocity"=2, "Current"=3, "Follower"=5, "MotionProfile"=6, "MotionMagic"=7, "MotionProfileArc"=10, "Disabled"=15] ("Control Mode")
        w1459 = T13 0 items=["PercentOutput"=0, "Position"=1, "Velocity"=2, "Current"=3, "Follower"=5, "MotionProfile"=6, "MotionMagic"=7, "MotionProfileArc"=10, "Disabled"=15] ("Control Mode")
        # "-0.186"
        # "-0.944"
        # ".135"
        n409 = call "Drive_Vi.vi"("Middle Thumb"=FALSE, "Z"=0.0, "Y"=-0.75, "X"=0.0) -> ()  [unwired: 8 in]
        n410 = call <vilib>:"CTRE_Phoenix_MotorControl_Set.vi"("error in (no error)"=w1442, "Output"=1.0, "Control Mode"=w1458, "PhoenixMotorControlDevRef"=w1443) -> ("error out"=w1438:errorcluster, "PhoenixMotorControlDevRef"=w1439:T9)  [unwired: 6 in]
        n411 = call <vilib>:"CTRE_Phoenix_MotorControl_Set.vi"("error in (no error)"=w1440, "Output"=0.0, "Control Mode"=w1459, "PhoenixMotorControlDevRef"=w1441) -> ("error out"=w1436:errorcluster, "PhoenixMotorControlDevRef"=w1437:T9)  [unwired: 6 in]
        n412 = Greater?(x=w1454, y=3) -> (0:w1453:bool)
        n413 = Wait (ms)(milliseconds to wait=u32 116) -> ()  [unwired: 1 out]
        n414 = call-poly <vilib>:"NT Read Value.vi"("Default Value"=0.0, "Name"="/limelight-drtrain/ty") -> ("Numeric"=w1445:dbl)  [unwired: 8 in, 1 out]
        "Ty 18" <- w1445
        n415 = call "Shooter_Equation.vi"("Right Trigger"=0.0, "Ty"=w1445) -> ()  [unwired: 10 in]
      }
      n416 = while {
        tunnel: w1243 -> [w1427]
        tunnel: w1242 -> [w1426]
        tunnel: w1241 -> [w1425]
        tunnel: w1240 -> [w1424]
        tunnel: [w1419] -> w1239
        tunnel: [w1418] -> w1238
        tunnel: [w1417] -> w1237
        tunnel: [w1416] -> w1236
        i -> [w1421]
        stop <- w1420 stop-if-true
        w1434 = T13 0 items=["PercentOutput"=0, "Position"=1, "Velocity"=2, "Current"=3, "Follower"=5, "MotionProfile"=6, "MotionMagic"=7, "MotionProfileArc"=10, "Disabled"=15] ("Control Mode")
        w1435 = T13 0 items=["PercentOutput"=0, "Position"=1, "Velocity"=2, "Current"=3, "Follower"=5, "MotionProfile"=6, "MotionMagic"=7, "MotionProfileArc"=10, "Disabled"=15] ("Control Mode")
        # "-0.186"
        # "-0.944"
        # ".135"
        n417 = call <vilib>:"CTRE_Phoenix_MotorControl_Set.vi"("error in (no error)"=w1426, "Output"=1.0, "Control Mode"=w1434, "PhoenixMotorControlDevRef"=w1427) -> ("error out"=w1418:errorcluster, "PhoenixMotorControlDevRef"=w1419:T9)  [unwired: 6 in]
        n418 = call <vilib>:"CTRE_Phoenix_MotorControl_Set.vi"("error in (no error)"=w1424, "Output"=0.0, "Control Mode"=w1435, "PhoenixMotorControlDevRef"=w1425) -> ("error out"=w1416:errorcluster, "PhoenixMotorControlDevRef"=w1417:T9)  [unwired: 6 in]
        n419 = call "Drive_Vi.vi"("Middle Thumb"=FALSE, "Z"=0.0, "Y"=0.0, "X"=0.0) -> ()  [unwired: 8 in]
        n420 = Greater?(x=w1421, y=35) -> (0:w1420:bool)
        n421 = call-poly <vilib>:"NT Read Value.vi"("Default Value"=0.0, "Name"="/limelight-drtrain/ty") -> ("Numeric"=w1429:dbl)  [unwired: 8 in, 1 out]
        "Ty 19" <- w1429
        n422 = Wait (ms)(milliseconds to wait=u32 100) -> ()  [unwired: 1 out]
        n423 = call "Shooter_Equation.vi"("Right Trigger"=0.0, "Ty"=w1429) -> ()  [unwired: 10 in]
      }
      n424 = while {
        tunnel: w1239 -> [w1399]
        tunnel: w1238 -> [w1398]
        tunnel: w1237 -> [w1397]
        tunnel: w1236 -> [w1396]
        tunnel: [w1391] -> w1235
        tunnel: [w1390] -> w1234
        tunnel: [w1389] -> w1233
        tunnel: [w1388] -> w1232
        tunnel: w1212 -> [w1382]
        tunnel: w1211 -> [w1383]
        tunnel: [w1383] -> w1210
        tunnel: [w1382] -> w1209
        i -> [w1393]
        stop <- w1392 stop-if-true
        w1410 = T13 0 items=["PercentOutput"=0, "Position"=1, "Velocity"=2, "Current"=3, "Follower"=5, "MotionProfile"=6, "MotionMagic"=7, "MotionProfileArc"=10, "Disabled"=15] ("Control Mode")
        w1411 = T13 0 items=["PercentOutput"=0, "Position"=1, "Velocity"=2, "Current"=3, "Follower"=5, "MotionProfile"=6, "MotionMagic"=7, "MotionProfileArc"=10, "Disabled"=15] ("Control Mode")
        # "-0.186"
        # "-0.944"
        # ".135"
        n425 = call "Turret_Aim.vi"("View Button"=FALSE, "Left Trigger"=0.0, "Orange Limit Pressed"=w1382, "Blue Limit Pressed"=w1383, "Right Bumper"=FALSE, "Left Bumper"=FALSE) -> ()  [unwired: 6 in]
        n426 = call "Drive_Vi.vi"("Middle Thumb"=FALSE, "Z"=0.0, "Y"=0.75, "X"=0.0) -> ()  [unwired: 8 in]
        n427 = call <vilib>:"CTRE_Phoenix_MotorControl_Set.vi"("error in (no error)"=w1398, "Output"=1.0, "Control Mode"=w1410, "PhoenixMotorControlDevRef"=w1399) -> ("error out"=w1390:errorcluster, "PhoenixMotorControlDevRef"=w1391:T9)  [unwired: 6 in]
        n428 = call <vilib>:"CTRE_Phoenix_MotorControl_Set.vi"("error in (no error)"=w1396, "Output"=-0.1, "Control Mode"=w1411, "PhoenixMotorControlDevRef"=w1397) -> ("error out"=w1388:errorcluster, "PhoenixMotorControlDevRef"=w1389:T9)  [unwired: 6 in]
        n429 = Greater?(x=w1393, y=5) -> (0:w1392:bool)
        n430 = Wait (ms)(milliseconds to wait=u32 50) -> ()  [unwired: 1 out]
        n431 = call-poly <vilib>:"NT Read Value.vi"("Default Value"=0.0, "Name"="/limelight-drtrain/ty") -> ("Numeric"=w1401:dbl)  [unwired: 8 in, 1 out]
        "Ty 20" <- w1401
        n432 = call "Shooter_Equation.vi"("Right Trigger"=0.0, "Ty"=w1401) -> ()  [unwired: 10 in]
      }
      n433 = while {
        tunnel: w1235 -> [w1369]
        tunnel: [w1362] -> _
        tunnel: w1233 -> [w1368]
        tunnel: w1232 -> [w1367]
        tunnel: w1234 -> [w1362]
        tunnel: [w1361] -> w1215
        tunnel: [w1360] -> w1214
        tunnel: [w1359] -> w1220
        tunnel: [w1358] -> w1218
        tunnel: w1210 -> [w1354]
        tunnel: w1209 -> [w1353]
        i -> [w1364]
        stop <- w1363 stop-if-true
        (unwired) FALSE ("Orange Limit Pressed")
        w1380 = T13 0 items=["PercentOutput"=0, "Position"=1, "Velocity"=2, "Current"=3, "Follower"=5, "MotionProfile"=6, "MotionMagic"=7, "MotionProfileArc"=10, "Disabled"=15] ("Control Mode")
        w1381 = T13 0 items=["PercentOutput"=0, "Position"=1, "Velocity"=2, "Current"=3, "Follower"=5, "MotionProfile"=6, "MotionMagic"=7, "MotionProfileArc"=10, "Disabled"=15] ("Control Mode")
        # "-0.186"
        # "-0.944"
        # ".135"
        n434 = call "Turret_Aim.vi"("View Button"=FALSE, "Left Trigger"=2.0, "Orange Limit Pressed"=w1353, "Blue Limit Pressed"=w1354, "Right Bumper"=FALSE, "Left Bumper"=FALSE) -> ()  [unwired: 6 in]
        n435 = call "Drive_Vi.vi"("Middle Thumb"=FALSE, "Z"=0.0, "Y"=-0.1, "X"=0.0) -> ()  [unwired: 8 in]
        n436 = call <vilib>:"CTRE_Phoenix_MotorControl_Set.vi"("error in (no error)"=w1362, "Output"=0.0, "Control Mode"=w1380, "PhoenixMotorControlDevRef"=w1369) -> ("error out"=w1358:errorcluster, "PhoenixMotorControlDevRef"=w1359:T9)  [unwired: 6 in]
        n437 = call <vilib>:"CTRE_Phoenix_MotorControl_Set.vi"("error in (no error)"=w1367, "Output"=-0.35, "Control Mode"=w1381, "PhoenixMotorControlDevRef"=w1368) -> ("error out"=w1361:errorcluster, "PhoenixMotorControlDevRef"=w1360:T9)  [unwired: 6 in]
        n438 = Greater?(x=w1364, y=10) -> (0:w1363:bool)
        n439 = Wait (ms)(milliseconds to wait=u32 100) -> ()  [unwired: 1 out]
        n440 = call-poly <vilib>:"NT Read Value.vi"("Default Value"=0.0, "Name"="/limelight-drtrain/ty") -> ("Numeric"=w1371:dbl)  [unwired: 8 in, 1 out]
        "Ty 21" <- w1371
        n441 = call "Shooter_Equation.vi"("Right Trigger"=2.0, "Ty"=w1371) -> ()  [unwired: 10 in]
      }
      n442 = while {
        tunnel: [w1297] -> w1219
        tunnel: w1220 -> [w1297]
        tunnel: [w1296] -> w1217
        tunnel: w1218 -> [w1296]
        tunnel: [w1295] -> w1216
        tunnel: w1215 -> [w1295]
        tunnel: [w1294] -> w1213
        tunnel: w1214 -> [w1294]
        i -> [w1287]
        stop <- w1286 stop-if-true
        n443 = Greater?(x=w1287, y=4) -> (0:w1286:bool)
        n444 = call "Drive_Vi.vi"("Middle Thumb"=TRUE, "Z"=0.15, "Y"=0.0, "X"=0.0) -> ()  [unwired: 8 in]
        n445 = Wait (ms)(milliseconds to wait=u32 100) -> ()  [unwired: 1 out]
      }
      n446 = while {
        tunnel: w1219 -> [w1339]
        tunnel: w1217 -> [w1332]
        tunnel: w1213 -> [w1338]
        tunnel: w1216 -> [w1337]
        i -> [w1334]
        stop <- w1333 stop-if-true
        w1350 = T13 0 items=["PercentOutput"=0, "Position"=1, "Velocity"=2, "Current"=3, "Follower"=5, "MotionProfile"=6, "MotionMagic"=7, "MotionProfileArc"=10, "Disabled"=15] ("Control Mode")
        w1351 = T13 0 items=["PercentOutput"=0, "Position"=1, "Velocity"=2, "Current"=3, "Follower"=5, "MotionProfile"=6, "MotionMagic"=7, "MotionProfileArc"=10, "Disabled"=15] ("Control Mode")
        # "-0.186"
        # "-0.944"
        # ".135"
        n447 = call "Drive_Vi.vi"("Middle Thumb"=FALSE, "Z"=0.0, "Y"=0.0, "X"=0.0) -> ()  [unwired: 8 in]
        n448 = call <vilib>:"CTRE_Phoenix_MotorControl_Set.vi"("error in (no error)"=w1332, "Output"=0.0, "Control Mode"=w1350, "PhoenixMotorControlDevRef"=w1339) -> ()  [unwired: 6 in, 2 out]
        n449 = call <vilib>:"CTRE_Phoenix_MotorControl_Set.vi"("error in (no error)"=w1337, "Output"=0.0, "Control Mode"=w1351, "PhoenixMotorControlDevRef"=w1338) -> ()  [unwired: 6 in, 2 out]
        n450 = Greater?(x=w1334, y=20) -> (0:w1333:bool)
        n451 = Wait (ms)(milliseconds to wait=u32 100) -> ()  [unwired: 1 out]
        n452 = call-poly <vilib>:"NT Read Value.vi"("Default Value"=0.0, "Name"="/limelight-drtrain/ty") -> ("Numeric"=w1341:dbl)  [unwired: 8 in, 1 out]
        "Ty 22" <- w1341
        n453 = call "Shooter_Equation.vi"("Right Trigger"=0.0, "Ty"=w1341) -> ()  [unwired: 10 in]
      }
    }
    frame "Angle Test" {
      n454 = call <vilib>:"CTRE_Phoenix_MotorControl_RefNumRegistryGet.vi"("refnum name"="Orange Back Turn") -> ("error out"=w1639:errorcluster, "PhoenixMotorControlDevRef"=w1640:T9)  [unwired: 9 in]
      n455 = call <vilib>:"CTRE_Phoenix_MotorControl_RefNumRegistryGet.vi"("refnum name"="Orange Back Drive") -> ("error out"=w1637:errorcluster, "PhoenixMotorControlDevRef"=w1638:T9)  [unwired: 9 in]
      n456 = while {
        tunnel: w1640 -> [w1683]
        tunnel: w1639 -> [w1681]
        tunnel: w1638 -> [w1676]
        tunnel: w1637 -> [w1675]
        tunnel: [w1672] -> w1634
        tunnel: [w1671] -> w1633
        tunnel: [w1670] -> w1632
        tunnel: [w1669] -> w1631
        i -> [w1686]
        stop <- w1684 stop-if-true
        w1673 = T13 0 items=["PercentOutput"=0, "Position"=1, "Velocity"=2, "Current"=3, "Follower"=5, "MotionProfile"=6, "MotionMagic"=7, "MotionProfileArc"=10, "Disabled"=15] ("Control Mode")
        w1678 = T13 0 items=["PercentOutput"=0, "Position"=1, "Velocity"=2, "Current"=3, "Follower"=5, "MotionProfile"=6, "MotionMagic"=7, "MotionProfileArc"=10, "Disabled"=15] ("Control Mode")
        n457 = call <vilib>:"CTRE_Phoenix_MotorControl_SetSelectedSensorPosition.vi"("error in (no error)"=w1681, "New Sensor Position"=0, "PhoenixMotorControlDevRef"=w1683) -> ("error out"=w1680:errorcluster, "PhoenixMotorControlDevRef"=w1682:T9)  [unwired: 7 in]
        n458 = Wait (ms)(milliseconds to wait=u32 20) -> ()  [unwired: 1 out]
        n459 = call <vilib>:"CTRE_Phoenix_MotorControl_Set.vi"("error in (no error)"=w1675, "Output"=0.0, "Control Mode"=w1673, "PhoenixMotorControlDevRef"=w1676) -> ("error out"=w1669:errorcluster, "PhoenixMotorControlDevRef"=w1670:T9)  [unwired: 6 in]
        n460 = call <vilib>:"CTRE_Phoenix_MotorControl_Set.vi"("error in (no error)"=w1680, "Output"=0.0, "Control Mode"=w1678, "PhoenixMotorControlDevRef"=w1682) -> ("error out"=w1671:errorcluster, "PhoenixMotorControlDevRef"=w1672:T9)  [unwired: 6 in]
        n461 = Greater?(x=w1686, y=u32 10) -> (0:w1684:bool)
      }
      n462 = while {
        tunnel: w1634 -> [w1657]
        tunnel: w1633 -> [w1658]
        tunnel: w1632 -> [w1662]
        tunnel: w1631 -> [w1661]
        tunnel: [w1656] -> w1630
        tunnel: [w1655] -> w1629
        tunnel: [w1654] -> w1628
        tunnel: [w1653] -> w1627
        i -> [w1667]
        stop <- w1665 stop-if-true
        w1659 = T13 0 items=["PercentOutput"=0, "Position"=1, "Velocity"=2, "Current"=3, "Follower"=5, "MotionProfile"=6, "MotionMagic"=7, "MotionProfileArc"=10, "Disabled"=15] ("Control Mode")
        w1664 = T13 1 items=["PercentOutput"=0, "Position"=1, "Velocity"=2, "Current"=3, "Follower"=5, "MotionProfile"=6, "MotionMagic"=7, "MotionProfileArc"=10, "Disabled"=15] ("Control Mode")
        n463 = Wait (ms)(milliseconds to wait=u32 20) -> ()  [unwired: 1 out]
        n464 = call <vilib>:"CTRE_Phoenix_MotorControl_Set.vi"("error in (no error)"=w1661, "Output"=0.0, "Control Mode"=w1659, "PhoenixMotorControlDevRef"=w1662) -> ("error out"=w1653:errorcluster, "PhoenixMotorControlDevRef"=w1654:T9)  [unwired: 6 in]
        n465 = call <vilib>:"CTRE_Phoenix_MotorControl_Set.vi"("error in (no error)"=w1658, "Output"=1024.0, "Control Mode"=w1664, "PhoenixMotorControlDevRef"=w1657) -> ("error out"=w1655:errorcluster, "PhoenixMotorControlDevRef"=w1656:T9)  [unwired: 6 in]
        n466 = Greater?(x=w1667, y=u32 10) -> (0:w1665:bool)
      }
      n467 = while {
        tunnel: w1630 -> [w1641]
        tunnel: w1629 -> [w1642]
        tunnel: w1628 -> [w1646]
        tunnel: w1627 -> [w1645]
        i -> [w1651]
        stop <- w1649 stop-if-true
        w1643 = T13 0 items=["PercentOutput"=0, "Position"=1, "Velocity"=2, "Current"=3, "Follower"=5, "MotionProfile"=6, "MotionMagic"=7, "MotionProfileArc"=10, "Disabled"=15] ("Control Mode")
        w1648 = T13 0 items=["PercentOutput"=0, "Position"=1, "Velocity"=2, "Current"=3, "Follower"=5, "MotionProfile"=6, "MotionMagic"=7, "MotionProfileArc"=10, "Disabled"=15] ("Control Mode")
        n468 = Wait (ms)(milliseconds to wait=u32 20) -> ()  [unwired: 1 out]
        n469 = call <vilib>:"CTRE_Phoenix_MotorControl_Set.vi"("error in (no error)"=w1645, "Output"=-0.1, "Control Mode"=w1643, "PhoenixMotorControlDevRef"=w1646) -> ()  [unwired: 6 in, 2 out]
        n470 = call <vilib>:"CTRE_Phoenix_MotorControl_Set.vi"("error in (no error)"=w1642, "Output"=0.0, "Control Mode"=w1648, "PhoenixMotorControlDevRef"=w1641) -> ()  [unwired: 6 in, 2 out]
        n471 = Greater?(x=w1651, y=u32 10) -> (0:w1649:bool)
      }
    }
  }
